vi "Main.vi"() -> ()   [LabVIEW 2017]
doc: "The myRIO Project template acquires acceleration data from the onboard accelerometer and displays the changes of acceleration values in a waveform chart."
uses:
  <vilib>/myRIO/Instrument Drivers/Onboard IO/DIO/typedefs/DIO Reference.ctl
  <vilib>/myRIO/Common/Instrument Driver Framework/Utilities/typedefs/myRIO Generic Hardware Reference.ctl
  <vilib>/myRIO/Common/Instrument Driver Framework/Utilities/typedefs/Hardware Version Enum.ctl
  <vilib>/myRIO/Common/Instrument Driver Framework/Utilities/typedefs/myRIO v1.0 Reference.ctl
  <vilib>/myRIO/Common/Instrument Driver Framework/Utilities/typedefs/Generic FPGA Reference.ctl
  <vilib>/myRIO/Common/Instrument Driver Framework/myRIO v1.0/DIO/typedefs/DIO Channels List.ctl
  <vilib>/myRIO/Common/Instrument Driver Framework/myRIO v1.0/DIO/typedefs/DIO Channels Enum.ctl
  <vilib>/userdefined/High Color/nirio_resource_hc.ctl
  <vilib>/myRIO/Common/Instrument Driver Framework/Utilities/vis/Is FPGA Ref Available.vi
  <vilib>/myRIO/Common/Instrument Driver Framework/myRIO v1.0/DIO/vis/myRIO v1.1 Open DIO.vi
  <vilib>/myRIO/Instrument Drivers/Onboard IO/DIO/vis/Read.vi
  <vilib>/myRIO/Instrument Drivers/Onboard IO/DIO/vis/Write.vi
  <vilib>/myRIO/Common/Instrument Driver Framework/Utilities/vis/Validate Channels.vi
  <vilib>/myRIO/Common/Instrument Driver Framework/myRIO v1.0/DIO/vis/myRIO v1.0 Reserve DIO.vi
  <vilib>/myRIO/Common/Instrument Driver Framework/myRIO v1.0/Resource Manager/vis/myRIO v1.0 Reserve Channel List.vi
  <vilib>/myRIO/Common/Instrument Driver Framework/myRIO v1.0/DIO/vis/myRIO v1.0 Build MUX Configuration DIO.vi
  <vilib>/myRIO/Common/Instrument Driver Framework/myRIO v1.0/Resource Manager/vis/myRIO v1.0 Reserve Channel.vi
  <vilib>/myRIO/Common/Instrument Driver Framework/myRIO v1.0/Resource Manager/vis/myRIO v1.0 Unreserve Channel.vi
  <vilib>/myRIO/Common/Instrument Driver Framework/myRIO v1.0/Resource Manager/vis/myRIO v1.0 Create Configuration List.vi
  <vilib>/myRIO/Common/Instrument Driver Framework/myRIO v1.0/Resource Manager/vis/myRIO v1.0 Build Mutex Name.vi
  GlobalVar.vi
  <vilib>/Utility/VariantDataType/GetNumericInfo.vi
  <vilib>/Utility/error.llb/Error Cluster From Error Code.vi
  <vilib>/myRIO/Common/Instrument Driver Framework/myRIO v1.0/myRIO v1.1 Open.vi
  <vilib>/myRIO/Common/Instrument Driver Framework/Utilities/vis/IO Manager.vi
  <vilib>/myRIO/Common/Instrument Driver Framework/Utilities/vis/Configuration Manager.vi
  <vilib>/myRIO/Common/Instrument Driver Framework/myRIO v1.0/Resource Manager/vis/myRIO v1.0 Configure IO.vi
  <vilib>/myRIO/Common/Instrument Driver Framework/myRIO v1.0/myRIO v1.0 Close.vi
  <vilib>/myRIO/Common/Instrument Driver Framework/myRIO v1.0/DIO/vis/myRIO v1.0 Write DIO.vi
  <vilib>/myRIO/Common/Instrument Driver Framework/myRIO v1.0/DIO/vis/myRIO v1.0 Read DIO.vi
  <vilib>/myRIO/Express VI/Onboard Devices/LED/LED Express VI.xnode
  <vilib>/myRIO/Instrument Drivers/Onboard IO/DIO/vis/myRIO DIO Open.xnode
  <vilib>/myRIO/Express VI/Onboard Devices/Button/Button Express VI.xnode
  <vilib>/myRIO/Instrument Drivers/Onboard IO/DIO/DIO.lvlib
panel:
  out "s? t:f":u32
  in  "servo3 drop_inBack 2":u8
  in  "servo3 pick_front 2":u8=45
  in  "start_seri 2":bool
  in  "done_servo_positioning 2":bool
  in  "inner_b_ir 2":dbl
  in  "inner_f_ir 2":dbl
  in  "target_ir_l 2":dbl
  in  "target_ir_r 2":dbl
  in  "start_cari 2":bool
  in  "done_positioning 2":bool
  in  "servo 3 dropfront 2":u8
  in  "servo 3 pickBack 2":u8
  in  "start_pick 2":bool
  in  "done_pickup 2":bool
  in  "D 2":dbl
  in  "Enum 2":enum16{"hold", "f", "b"}(ring)
  in  "trun 2":bool
  out "binary 2":u32
  out "MOTOR_POW":i8
  in  "Enum":enum16{"hold", "f", "b"}(ring)
  in  "D":dbl
  out "binary":u32
  in  "trun":bool
  in  "servo 3 dropfront":u8
  in  "servo 3 pickBack":u8
  in  "start_pick":bool
  in  "done_pickup":bool
  in  "servo3 pick_front":u8=45
  in  "servo3 drop_inBack":u8
  in  "done_servo_positioning":bool
  in  "start_seri":bool
  in  "inner_f_ir":dbl
  in  "inner_b_ir":dbl
  in  "target_ir_r":dbl
  in  "target_ir_l":dbl
  in  "done_positioning":bool
  in  "start_cari":bool
  in  "x":dbl
  in  "start_step_for_takePic":bool
  in  "Stop (F)":bool
  out "Image Out":T1(plugin-control)
  in  "Carzeta":dbl
  in  "start_rotate_for_takePic":bool
  out "L_MOTOR_POS":i32
  out "R_MOTOR_POS":i32
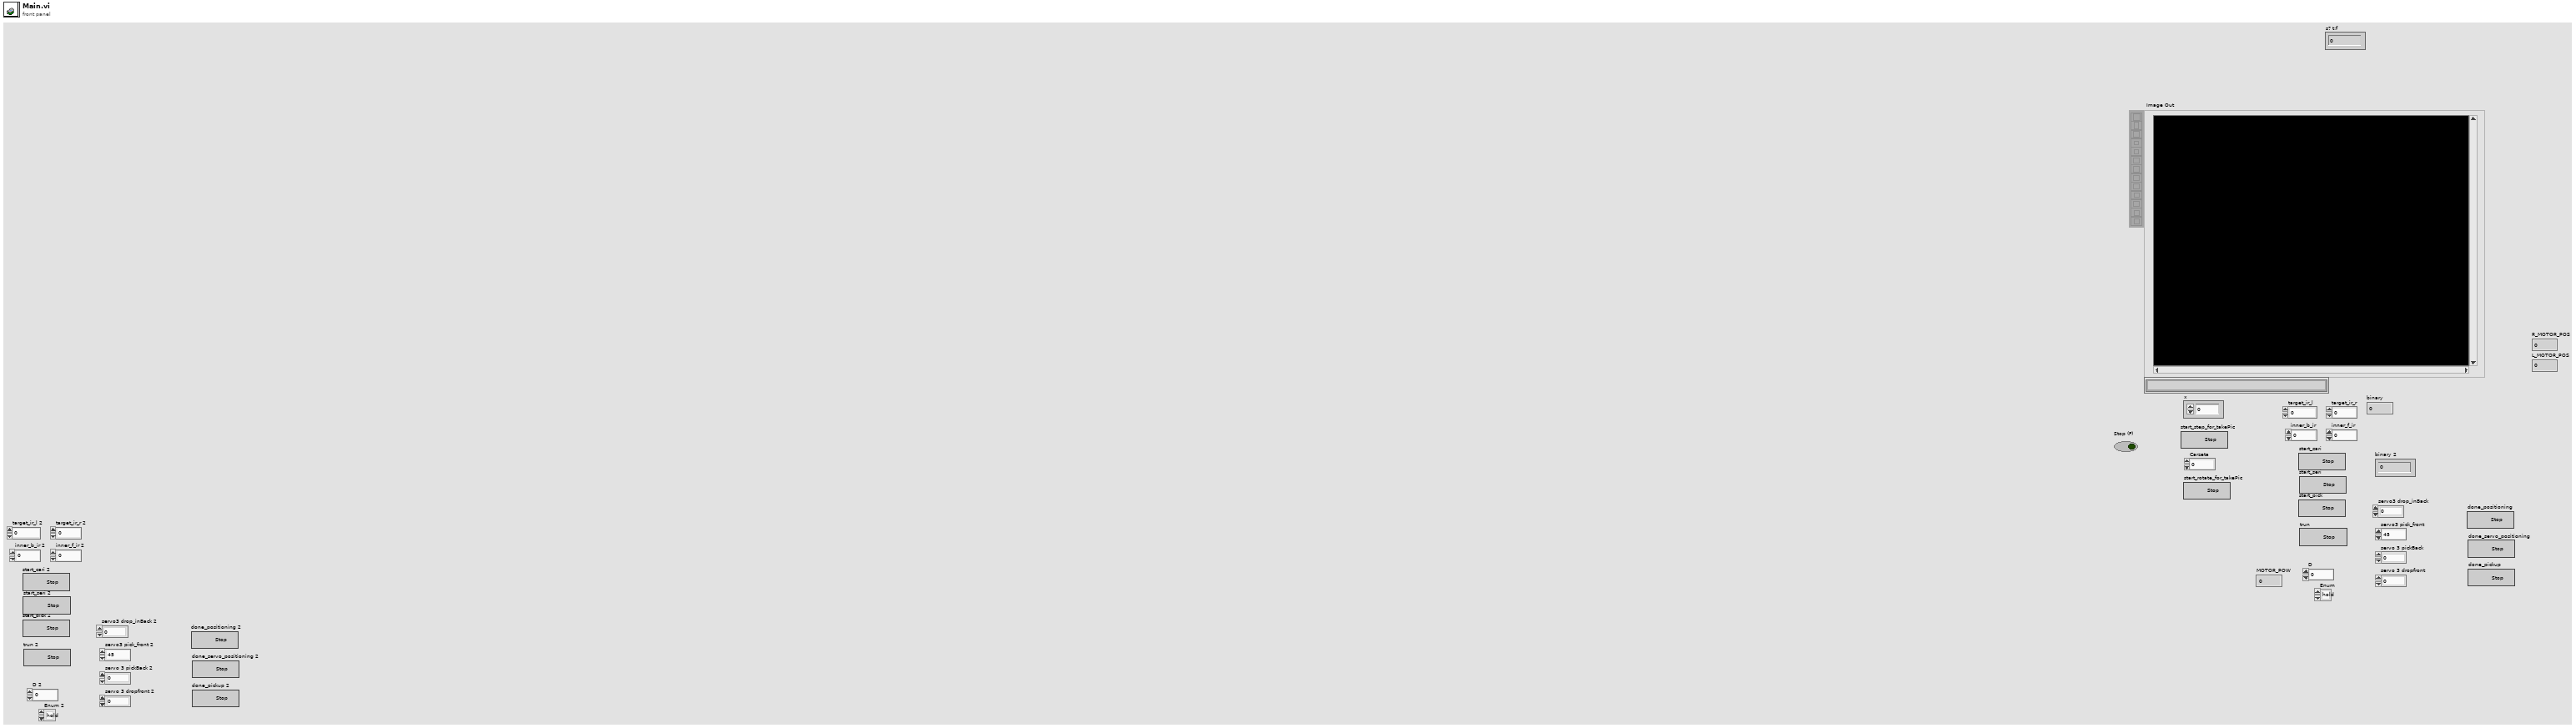
[diagram p1: front panel]
types:
  T1 = typedef "IMAQ Image.ctl" = refnum<image>
  T2 = typedef "DIO.lvlib/DIO Reference.ctl" = cluster{"myRIO Reference":T3, "DIO Channels List":T7}
  T3 = typedef "myRIO Generic Hardware Reference.ctl" = cluster{"myRIO Model":T4, "myRIO Hardware Reference":T5}
  T4 = typedef "Hardware Version Enum.ctl" = enum16{"Unknown", "myRIO-1900", "myRIO-1950", "roboRIO", "NI ELVIS RIO CM"}
  T5 = typedef "myRIO v1.0 Reference.ctl" = cluster{"Generic FPGA Reference":T6, "Allow multiple opens":bool}
  T6 = typedef "Generic FPGA Reference.ctl" = refnum<k20>
  T7 = typedef "DIO Channels List.ctl" = T8[]
  T8 = typedef "DIO Channels Enum.ctl" = enum16{"Not Connected", "C/DIO0", "C/DIO1", "C/DIO2", "C/DIO3", "C/DIO4", "C/DIO5", "C/DIO6", "C/DIO7", "A/DIO0", "A/DIO1", "A/DIO2", "A/DIO3", "A/DIO4", "A/DIO5", "A/DIO6", "A/DIO7", "A/DIO8", "A/DIO9", "A/DIO10", "A/DIO11", "A/DIO12", "A/DIO13", "A/DIO14", "A/DIO15", "B/DIO0", "B/DIO1", "B/DIO2", "B/DIO3", "B/DIO4", "B/DIO5", "B/DIO6", "B/DIO7", "B/DIO8", "B/DIO9", "B/DIO10", "B/DIO11", "B/DIO12", "B/DIO13", "B/DIO14", "B/DIO15", "LED0", "LED1", "LED2", "LED3", "Button0", "DIO/DIO0", "DIO/DIO1", "DIO/DIO2", "DIO/DIO3", "DIO/DIO4", "DIO/DIO5", "DIO/DIO6", "DIO/DIO7", "DIO/DIO8", "DIO/DIO9", "SPI/CS0", "SPI/CS1", "SPI/CS2", "SPI/CS3", "LED RADIO (Green)", "LED RADIO (Red)", "LED COMM (Green)", "LED COMM (Red)", "LED MODE (Green)", "LED MODE (Red)"}
  T9 = typedef "nirio_resource_hc.ctl" = tag
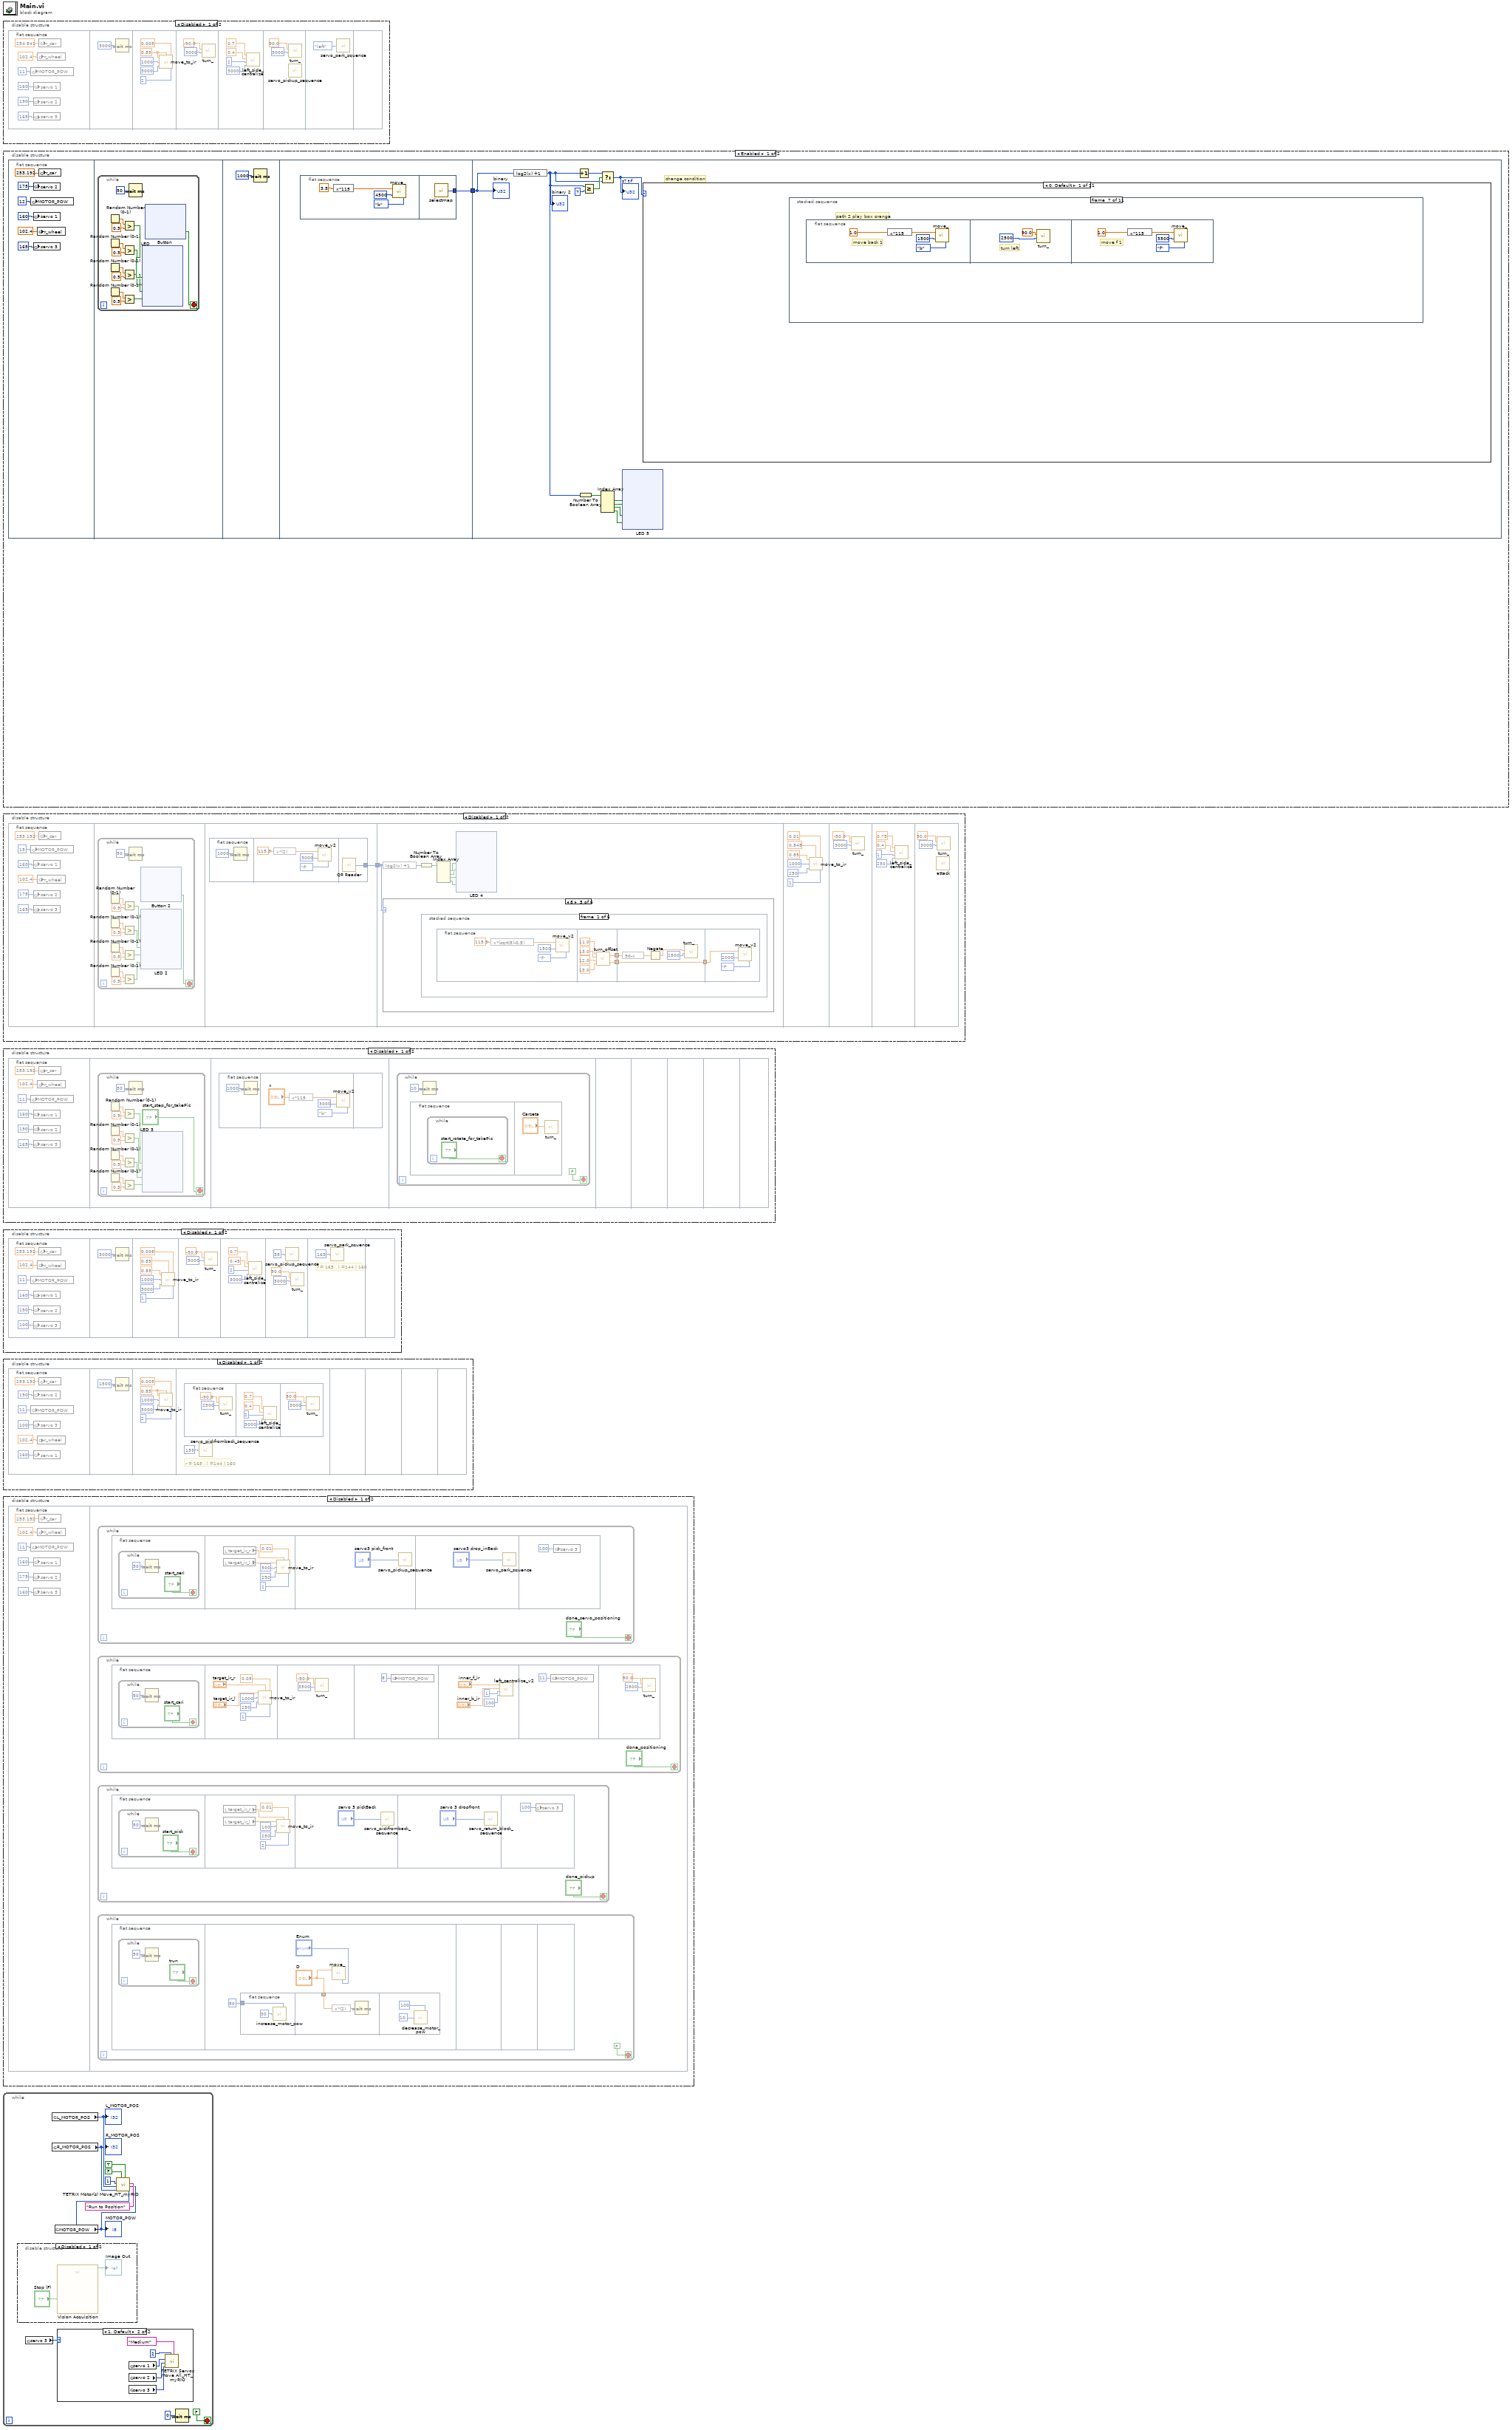
[diagram p0: block diagram]
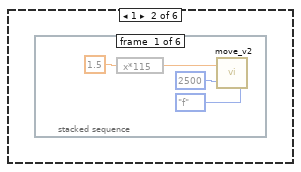
[diagram p5: hidden frame]
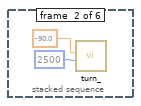
[diagram p6: hidden frame]
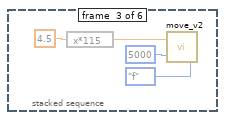
[diagram p7: hidden frame]
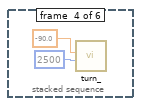
[diagram p8: hidden frame]
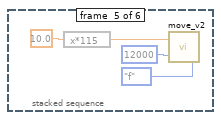
[diagram p9: hidden frame]
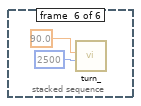
[diagram p10: hidden frame]
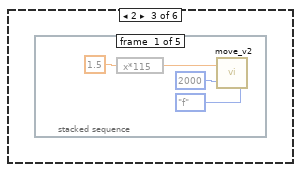
[diagram p11: hidden frame]
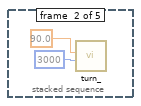
[diagram p12: hidden frame]
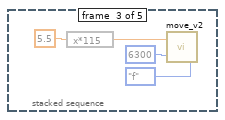
[diagram p13: hidden frame]
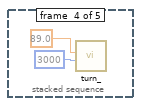
[diagram p14: hidden frame]
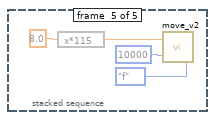
[diagram p15: hidden frame]
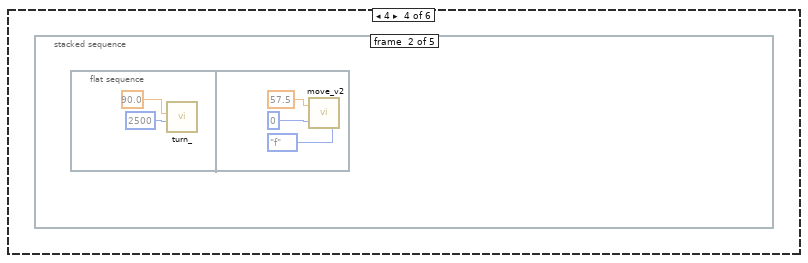
[diagram p16: hidden frame]
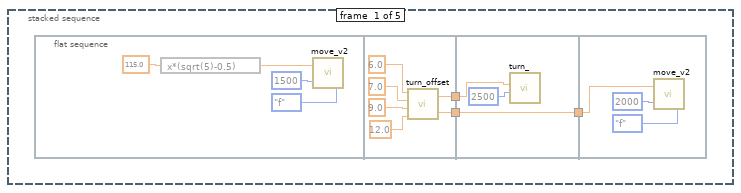
[diagram p17: hidden frame]
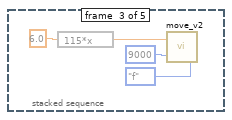
[diagram p18: hidden frame]
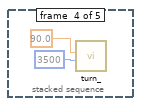
[diagram p19: hidden frame]
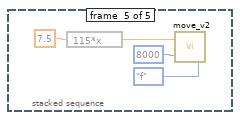
[diagram p20: hidden frame]
diagram:
  n1 = disable-structure shown="Disabled" {
    frame Disabled {
      n2 = flat-sequence {
        frame #0 {
          n3 = global write "GlobalVar.vi" "MOTOR_POW"(i8 11 ("MOTOR_POW")) -> ()
          n4 = global write "GlobalVar.vi" "servo 1"(u8 160 ("servo 1")) -> ()
          n5 = global write "GlobalVar.vi" "servo 2"(u8 190 ("servo 2")) -> ()
          n6 = global write "GlobalVar.vi" "servo 3"(u8 165 ("servo 3")) -> ()
          n7 = global write "GlobalVar.vi" "r_wheel"(102.4 ("r_wheel")) -> ()
          n8 = global write "GlobalVar.vi" "r_car"(254.841 ("r_car")) -> ()
        }
        frame #1 {
          n9 = Wait (ms)(milliseconds to wait=u32 3000) -> ()  [unwired: 1 out]
        }
        frame #2 {
          w12 = 0.85 ("target_ir_r")
          n10 = call "move_to_ir.vi"("step"=2, "precision"=0.005, "target_ir_r"=w12, "samples"=3000, "delay_after"=u32 1000, "target_ir_l"=w12) -> ()
        }
        frame #3 {
          n11 = call "turn_.vi"("delay"=u32 3000, "Carzeta"=-90.0) -> ()  [unwired: 10 in]
        }
        frame #4 {
          n12 = call "left_side_centralize.vi"("samples"=3000, "step(mm)"=2, "inner_b_ir"=0.4, "inner_f_ir"=0.7) -> ()
        }
        frame #5 {
          n13 = call "servo_pickup_sequence.vi"() -> ()  [unwired: 12 in]
          n14 = call "turn_.vi"("delay"=u32 3000, "Carzeta"=90.0) -> ()  [unwired: 10 in]
        }
        frame #6 {
          n15 = call "servo_park_squence.vi"("servo 3"=enum16{"left", "right"}."left" ("pos")) -> ()
        }
        frame #7 {
        }
      }
    }
    frame Enabled {
    }
  }
  n16 = disable-structure shown="Enabled" {
    frame Enabled {
      n17 = flat-sequence {
        tunnel: [w117] -> w22
        tunnel: w22 -> [w128]
        frame #0 {
          n18 = global write "GlobalVar.vi" "MOTOR_POW"(i8 12 ("MOTOR_POW")) -> ()
          n19 = global write "GlobalVar.vi" "servo 2"(u8 175 ("servo 2")) -> ()
          n20 = global write "GlobalVar.vi" "servo 1"(u8 160 ("servo 1")) -> ()
          n21 = global write "GlobalVar.vi" "servo 3"(u8 165 ("servo 3")) -> ()
          n22 = global write "GlobalVar.vi" "r_wheel"(102.4 ("r_wheel")) -> ()
          n23 = global write "GlobalVar.vi" "r_car"(253.192 ("r_car")) -> ()
        }
        frame #1 {
          n24 = while {
            stop <- w29 stop-if-true
            n25 = Random Number (0-1)() -> (number: 0 to 1=w34:dbl)
            n26 = Random Number (0-1)() -> (number: 0 to 1=w41:dbl)
            n27 = Random Number (0-1)() -> (number: 0 to 1=w38:dbl)
            n28 = Random Number (0-1)() -> (number: 0 to 1=w37:dbl)
            n29 = Greater?(x=w34, y=0.5) -> (0:w33:bool)
            n30 = Greater?(x=w41, y=0.5) -> (0:w32:bool)
            n31 = Greater?(x=w38, y=0.5) -> (0:w31:bool)
            n32 = Greater?(x=w37, y=0.5) -> (0:w30:bool)
            n33 = Wait (ms)(milliseconds to wait=u32 50) -> ()  [unwired: 1 out]
            n34 = xnode "LED"("LED0"=w33, "LED1"=w32, "LED2"=w31, "LED3"=w30) -> ()  [unwired: 1 in, 1 out]
            n35 = xnode "Button"() -> ("Value"=w29:bool)  [unwired: 1 in, 1 out]
          }
        }
        frame #2 {
          n36 = Wait (ms)(milliseconds to wait=u32 1000) -> ()  [unwired: 1 out]
        }
        frame #3 {
          n37 = flat-sequence {
            tunnel: [w122] -> w117
            frame #0 {
              n38 = expression code="x*115"(3.5 ("x")) -> (w120:dbl)
              n39 = call "move_.vi"("Enum"=enum16{"hold", "f", "b"}."b", "delay"=u32 4500, "D"=w120) -> ()  [unwired: 1 in]
            }
            frame #1 {
              n40 = call "selectmap.vi"() -> ("binary"=w122:u32)
            }
          }
        }
        frame #4 {
          # "change condition"
          n41 = expression code="log2(x) +1"(w128) -> (w124:u32)
          "binary 2" <- w124
          n42 = Increment(x=w124) -> (x+1=w125:u32)
          n43 = Number To Boolean Array(number=w124) -> (Boolean array=w133:bool[])
          n44 = Greater Or Equal?(x=w124, y=u32 7) -> (x >= y?=w126:bool)
          n45 = Select(t=w125, s=w126, f=w124) -> (s? t:f=w123:u32)
          "s? t:f" <- w123
          n46 = Index Array(array=w133) -> (element #1=w132:bool, element #2=w131:bool, element #3=w130:bool, element #4=w129:bool)  [unwired: 4 in]
          n47 = xnode "LED 5"("LED0"=w132, "LED1"=w131, "LED2"=w130, "LED3"=w129) -> ()  [unwired: 1 in, 1 out]
          n48 = case shown="0, Default" w123 {
            frame 0, Default {
              n49 = stacked-sequence {
                frame #0 {
                  # "font box bule"
                  n50 = flat-sequence {
                    frame #0 {
                      n51 = expression code="x*115"(1.5) -> (w175:dbl)
                      n52 = call "move_.vi"("Enum"=enum16{"hold", "f", "b"}."b", "delay"=u32 2500, "D"=w175) -> ()  [unwired: 1 in]
                    }
                    frame #1 {
                      n53 = call "turn_.vi"("delay"=u32 3000, "Carzeta"=90.0) -> ()  [unwired: 10 in]
                    }
                    frame #2 {
                      n54 = expression code="x*115"(5.0) -> (w181:dbl)
                      n55 = call "move_.vi"("Enum"=enum16{"hold", "f", "b"}."f", "delay"=u32 5500, "D"=w181) -> ()  [unwired: 1 in]
                    }
                    frame #3 {
                      n56 = call "turn_.vi"("delay"=u32 3000, "Carzeta"=-90.0) -> ()  [unwired: 10 in]
                    }
                    frame #4 {
                      n57 = expression code="x*115"(1.0) -> (w187:dbl)
                      n58 = call "move_.vi"("Enum"=enum16{"hold", "f", "b"}."f", "delay"=u32 2500, "D"=w187) -> ()  [unwired: 1 in]
                    }
                    frame #5 {
                      n59 = call "turn_.vi"("delay"=u32 3000, "Carzeta"=90.0) -> ()  [unwired: 10 in]
                    }
                  }
                }
                frame #1 {
                  # "play blue"
                  n60 = flat-sequence {
                    tunnel: [w193] -> w191
                    tunnel: [w192] -> w190
                    tunnel: w191 -> [w198]
                    tunnel: w190 -> [w197]
                    frame #0 {
                      w192 = 0.84 ("target_ir_l")
                      w193 = 0.84 ("target_ir_r")
                      n61 = call "integal_caribat_squence.vi"("inner_b_ir"=0.4, "inner_f_ir"=0.8, "target_ir_l"=w192, "target_ir_r"=w193, "precision"=0.008) -> ()
                    }
                    frame #1 {
                      n62 = call "integal_pickup_sequence .vi"("store_pos"=u8 156, "pick_pos"=u8 52, "target_ir_l"=w197, "target_ir_r"=w198, "precision"=0.05) -> ()
                    }
                  }
                }
                frame #2 {
                  # "move foward 2 box green"
                  n63 = flat-sequence {
                    frame #0 {
                      n64 = call "turn_.vi"("delay"=u32 5000, "Carzeta"=159.44) -> ()  [unwired: 10 in]
                    }
                    frame #1 {
                      n65 = expression code="x*115"(8.54) -> (w205:dbl)
                      n66 = call "move_v2.vi"("delay"=u32 2700, "Enum"=enum16{"hold", "f", "b"}."f", "D"=w205) -> ()  [unwired: 1 in]
                    }
                  }
                }
                frame #3 {
                  # "turn left 2 box green"
                  n67 = flat-sequence {
                    frame #0 {
                      n68 = call "turn_.vi"("delay"=u32 3300, "Carzeta"=110.56) -> ()  [unwired: 10 in]
                    }
                    frame #1 {
                      n69 = expression code="x*115"(8.0) -> (w212:dbl)
                      n70 = call "move_v2.vi"("delay"=u32 2500, "Enum"=enum16{"hold", "f", "b"}."f", "D"=w212) -> ()  [unwired: 1 in]
                    }
                    frame #2 {
                      n71 = call "turn_.vi"("delay"=u32 2500, "Carzeta"=-90.0) -> ()  [unwired: 10 in]
                    }
                  }
                }
                frame #4 {
                  # "play orange 2 right store"
                  n72 = flat-sequence {
                    tunnel: [w219] -> w217
                    tunnel: [w218] -> w216
                    tunnel: w217 -> [w224]
                    tunnel: w216 -> [w223]
                    frame #0 {
                      w218 = 0.84 ("target_ir_l")
                      w219 = 0.84 ("target_ir_r")
                      n73 = call "integal_caribat_squence.vi"("inner_b_ir"=0.4, "inner_f_ir"=0.8, "target_ir_l"=w218, "target_ir_r"=w219, "precision"=0.008) -> ()
                    }
                    frame #1 {
                      n74 = call "integal_pickup_sequence .vi"("store_pos"=u8 183, "pick_pos"=u8 52, "target_ir_l"=w223, "target_ir_r"=w224, "precision"=0.05) -> ()
                    }
                  }
                }
                frame #5 {
                  # "green 2 box green"
                  n75 = call "integal_return.vi"("servo 3 dropfront"=u8 52, "servo 3 pickBack"=u8 154) -> ()
                }
                frame #6 {
                  # "path 2 play box orange"
                  n76 = flat-sequence {
                    frame #0 {
                      # "move back 1"
                      n77 = expression code="x*115"(1.0) -> (w233:dbl)
                      n78 = call "move_.vi"("Enum"=enum16{"hold", "f", "b"}."b", "delay"=u32 1500, "D"=w233) -> ()  [unwired: 1 in]
                    }
                    frame #1 {
                      # "turn left"
                      n79 = call "turn_.vi"("delay"=u32 2500, "Carzeta"=90.0) -> ()  [unwired: 10 in]
                    }
                    frame #2 {
                      # "move f 1"
                      n80 = expression code="x*115"(1.0) -> (w239:dbl)
                      n81 = call "move_.vi"("Enum"=enum16{"hold", "f", "b"}."f", "delay"=u32 3500, "D"=w239) -> ()  [unwired: 1 in]
                    }
                  }
                }
                frame #7 {
                  # "pick red 2 store left"
                  n82 = flat-sequence {
                    tunnel: [w243] -> w241
                    tunnel: [w242] -> w240
                    tunnel: w241 -> [w248]
                    tunnel: w240 -> [w247]
                    frame #0 {
                      w242 = 0.84 ("target_ir_l")
                      w243 = 0.84 ("target_ir_r")
                      n83 = call "integal_caribat_squence.vi"("inner_b_ir"=0.4, "inner_f_ir"=0.8, "target_ir_l"=w242, "target_ir_r"=w243, "precision"=0.008) -> ()
                    }
                    frame #1 {
                      n84 = call "integal_pickup_sequence .vi"("store_pos"=u8 156, "pick_pos"=u8 52, "target_ir_l"=w247, "target_ir_r"=w248, "precision"=0.05) -> ()
                    }
                  }
                }
                frame #8 {
                  # "return orange 2 orange"
                  n85 = call "integal_return.vi"("servo 3 dropfront"=u8 52, "servo 3 pickBack"=u8 183) -> ()
                }
                frame #9 {
                  # "foward 2 parking"
                  n86 = flat-sequence {
                    frame #0 {
                      n87 = call "servo_pickfromback_sequence.vi"("pick_pos"=u8 154) -> ()
                    }
                    frame #1 {
                      n88 = global write "GlobalVar.vi" "servo 3"(u8 30 ("servo 3")) -> ()
                    }
                  }
                  n89 = flat-sequence {
                    frame #0 {
                      n90 = call "turn_.vi"("delay"=u32 5000, "Carzeta"=180.0) -> ()  [unwired: 10 in]
                    }
                    frame #1 {
                      n91 = expression code="x*115"(4.5) -> (w260:dbl)
                      n92 = call "move_.vi"("Enum"=enum16{"hold", "f", "b"}."f", "delay"=u32 5500, "D"=w260) -> ()  [unwired: 1 in]
                    }
                  }
                }
                frame #10 {
                  n93 = flat-sequence {
                    frame #0 {
                      n94 = call "turn_.vi"("delay"=u32 3000, "Carzeta"=-90.0) -> ()  [unwired: 10 in]
                    }
                    frame #1 {
                      n95 = expression code="x*115"(1.5) -> (w266:dbl)
                      n96 = call "move_.vi"("Enum"=enum16{"hold", "f", "b"}."f", "delay"=u32 3000, "D"=w266) -> ()  [unwired: 1 in]
                    }
                  }
                }
              }
            }
            frame 1 {
              n97 = stacked-sequence {
                frame #0 {
                  # "out parking"
                  n98 = flat-sequence {
                    tunnel: [w272] -> w270
                    tunnel: [w271] -> w268
                    tunnel: w270 -> [w279]
                    tunnel: [w278] -> w269
                    tunnel: w268 -> [w278]
                    tunnel: w269 -> [w281]
                    frame #0 {
                      n99 = call "turn_offset.vi"("x2"=17.0, "x1"=16.0, "y2"=16.0, "y1"=13.0) -> ("dis_"=w271:dbl, "zeta"=w272:dbl)
                    }
                    frame #1 {
                      n100 = expression code="-(45-x)"(w279) -> (w277:dbl)
                      n101 = call "turn_.vi"("delay"=u32 3000, "Carzeta"=w277) -> ()  [unwired: 10 in]
                    }
                    frame #2 {
                      n102 = call "move_.vi"("Enum"=enum16{"hold", "f", "b"}."b", "delay"=u32 2000, "D"=w281) -> ()  [unwired: 1 in]
                    }
                  }
                }
                frame #1 {
                  # "path 2 box blue"
                  n103 = flat-sequence {
                    frame #0 {
                      n104 = call "turn_.vi"("delay"=u32 3000, "Carzeta"=-90.0) -> ()  [unwired: 10 in]
                    }
                    frame #1 {
                      # "foward 2 blue"
                      n105 = expression code="x*115"(6.0) -> (w288:dbl)
                      n106 = call "move_.vi"("Enum"=enum16{"hold", "f", "b"}."f", "delay"=u32 6500, "D"=w288) -> ()  [unwired: 1 in]
                    }
                    frame #2 {
                      # "turn left"
                      n107 = call "turn_.vi"("delay"=u32 3000, "Carzeta"=90.0) -> ()  [unwired: 10 in]
                    }
                    frame #3 {
                      # "foward 2 blue"
                      n108 = expression code="x*115"(1.0) -> (w294:dbl)
                      n109 = call "move_.vi"("Enum"=enum16{"hold", "f", "b"}."f", "delay"=u32 1500, "D"=w294) -> ()  [unwired: 1 in]
                    }
                    frame #4 {
                      # "turn right"
                      n110 = call "turn_.vi"("delay"=u32 3000, "Carzeta"=-90.0) -> ()  [unwired: 10 in]
                    }
                  }
                }
                frame #2 {
                  # "keep yellow 2 left stored"
                  n111 = flat-sequence {
                    tunnel: [w301] -> w299
                    tunnel: [w300] -> w298
                    tunnel: w299 -> [w306]
                    tunnel: w298 -> [w305]
                    frame #0 {
                      w300 = 0.84 ("target_ir_l")
                      w301 = 0.84 ("target_ir_r")
                      n112 = call "integal_caribat_squence.vi"("inner_b_ir"=0.4, "inner_f_ir"=0.8, "target_ir_l"=w300, "target_ir_r"=w301, "precision"=0.008) -> ()
                    }
                    frame #1 {
                      n113 = call "integal_pickup_sequence .vi"("store_pos"=u8 156, "pick_pos"=u8 52, "target_ir_l"=w305, "target_ir_r"=w306, "precision"=0.05) -> ()
                    }
                  }
                }
                frame #3 {
                  # "path 2 box yellow(1)"
                  n114 = flat-sequence {
                    frame #0 {
                      # "turn right"
                      n115 = call "turn_.vi"("delay"=u32 5000, "Carzeta"=-142.125) -> ()  [unwired: 10 in]
                    }
                    frame #1 {
                      # "foward 2 yellow"
                      n116 = expression code="x*115"(11.4) -> (w313:dbl)
                      n117 = call "move_v2.vi"("delay"=u32 3500, "Enum"=enum16{"hold", "f", "b"}."f", "D"=w313) -> ()  [unwired: 1 in]
                    }
                    frame #2 {
                      # "turn right"
                      n118 = call "turn_.vi"("delay"=u32 2000, "Carzeta"=-37.875) -> ()  [unwired: 10 in]
                    }
                  }
                }
                frame #4 {
                  # "green 2 right stored"
                  n119 = flat-sequence {
                    tunnel: [w321] -> w319
                    tunnel: [w320] -> w318
                    tunnel: w319 -> [w326]
                    tunnel: w318 -> [w325]
                    frame #0 {
                      w320 = 0.84 ("target_ir_l")
                      w321 = 0.84 ("target_ir_r")
                      n120 = call "integal_caribat_squence.vi"("inner_b_ir"=0.4, "inner_f_ir"=0.8, "target_ir_l"=w320, "target_ir_r"=w321, "precision"=0.008) -> ()
                    }
                    frame #1 {
                      n121 = call "integal_pickup_sequence .vi"("store_pos"=u8 183, "pick_pos"=u8 52, "target_ir_l"=w325, "target_ir_r"=w326, "precision"=0.04) -> ()
                    }
                  }
                }
                frame #5 {
                  # "yellow 2 yellow"
                  # "154"
                  n122 = call "integal_return.vi"("servo 3 dropfront"=u8 52, "servo 3 pickBack"=u8 154) -> ()
                }
                frame #6 {
                  # "path 2 box green (1)"
                  n123 = flat-sequence {
                    frame #0 {
                      # "turn right"
                      n124 = call "turn_.vi"("delay"=u32 3000, "Carzeta"=-90.0) -> ()  [unwired: 10 in]
                    }
                    frame #1 {
                      # "forward 2 g"
                      n125 = expression code="x*115"(2.0) -> (w336:dbl)
                      n126 = call "move_.vi"("Enum"=enum16{"hold", "f", "b"}."f", "delay"=u32 2500, "D"=w336) -> ()  [unwired: 1 in]
                    }
                  }
                }
                frame #7 {
                  # "path 2 box green (2)"
                  n127 = flat-sequence {
                    frame #0 {
                      # "turn right"
                      n128 = call "turn_.vi"("delay"=u32 3000, "Carzeta"=-90.0) -> ()  [unwired: 10 in]
                    }
                    frame #1 {
                      # "foward 2 green"
                      n129 = expression code="x*115"(9.0) -> (w341:dbl)
                      n130 = call "move_v2.vi"("delay"=u32 3000, "Enum"=enum16{"hold", "f", "b"}."f", "D"=w341) -> ()  [unwired: 1 in]
                    }
                    frame #2 {
                      n131 = call "turn_.vi"("delay"=u32 3000, "Carzeta"=-90.0) -> ()  [unwired: 10 in]
                    }
                  }
                }
                frame #8 {
                  # "red 2 stored left"
                  n132 = flat-sequence {
                    tunnel: [w355] -> w347
                    tunnel: [w354] -> w346
                    tunnel: w347 -> [w360]
                    tunnel: w346 -> [w359]
                    frame #0 {
                      w354 = 0.84 ("target_ir_l")
                      w355 = 0.84 ("target_ir_r")
                      n133 = call "integal_caribat_squence.vi"("inner_b_ir"=0.4, "inner_f_ir"=0.8, "target_ir_l"=w354, "target_ir_r"=w355, "precision"=0.008) -> ()
                    }
                    frame #1 {
                      n134 = call "integal_pickup_sequence .vi"("store_pos"=u8 156, "pick_pos"=u8 52, "target_ir_l"=w359, "target_ir_r"=w360, "precision"=0.04) -> ()
                    }
                  }
                  n135 = disable-structure shown="Disabled" {
                    frame Disabled {
                      n136 = flat-sequence {
                        frame #0 {
                          n137 = call "integal_caribat_squence.vi"("inner_b_ir"=0.4, "inner_f_ir"=0.8, "target_ir_l"=0.84, "target_ir_r"=0.84, "precision"=0.008) -> ()
                        }
                        frame #1 {
                          n138 = call "servo_return_block_sequence.vi"("servo 3"=u8 52) -> ()
                        }
                      }
                    }
                    frame Enabled {
                    }
                  }
                }
                frame #9 {
                  # "path 2 parking"
                  n139 = flat-sequence {
                    frame #0 {
                      n140 = call "servo_pickfromback_sequence.vi"("pick_pos"=u8 182) -> ()
                    }
                    frame #1 {
                      n141 = global write "GlobalVar.vi" "servo 3"(u8 52 ("servo 3")) -> ()
                    }
                  }
                  n142 = flat-sequence {
                    frame #0 {
                      n143 = call "turn_.vi"("delay"=u32 3000, "Carzeta"=-90.0) -> ()  [unwired: 10 in]
                    }
                    frame #1 {
                      n144 = expression code="x*115"(7.0) -> (w370:dbl)
                      n145 = call "move_v2.vi"("delay"=u32 2300, "Enum"=enum16{"hold", "f", "b"}."f", "D"=w370) -> ()  [unwired: 1 in]
                    }
                    frame #2 {
                      n146 = call "turn_.vi"("delay"=u32 3000, "Carzeta"=-90.0) -> ()  [unwired: 10 in]
                    }
                    frame #3 {
                      n147 = expression code="x*115"(5.0) -> (w376:dbl)
                      n148 = call "move_.vi"("Enum"=enum16{"hold", "f", "b"}."f", "delay"=u32 4500, "D"=w376) -> ()  [unwired: 1 in]
                    }
                  }
                }
              }
            }
            frame 2 {
              n149 = stacked-sequence {
                frame #0 {
                  # "out parking"
                  n150 = flat-sequence {
                    tunnel: [w382] -> w380
                    tunnel: [w381] -> w378
                    tunnel: w380 -> [w389]
                    tunnel: [w388] -> w379
                    tunnel: w378 -> [w388]
                    tunnel: w379 -> [w391]
                    frame #0 {
                      n151 = call "turn_offset.vi"("x2"=5.0, "x1"=7.0, "y2"=9.0, "y1"=8.0) -> ("dis_"=w381:dbl, "zeta"=w382:dbl)
                    }
                    frame #1 {
                      n152 = expression code="-45-x"(w389) -> (w387:dbl)
                      n153 = call "turn_.vi"("delay"=u32 3000, "Carzeta"=w387) -> ()  [unwired: 10 in]
                    }
                    frame #2 {
                      n154 = call "move_.vi"("Enum"=enum16{"hold", "f", "b"}."b", "delay"=u32 2000, "D"=w391) -> ()  [unwired: 1 in]
                    }
                  }
                }
                frame #1 {
                  # "path 2 box green"
                  n155 = flat-sequence {
                    frame #0 {
                      # "turn left"
                      n156 = call "turn_.vi"("delay"=u32 3000, "Carzeta"=90.0) -> ()  [unwired: 10 in]
                    }
                    frame #1 {
                      n157 = expression code="x*115"(1.0) -> (w398:dbl)
                      n158 = call "move_.vi"("Enum"=enum16{"hold", "f", "b"}."b", "delay"=u32 3500, "D"=w398) -> ()  [unwired: 1 in]
                    }
                    frame #2 {
                      n159 = call "turn_.vi"("delay"=u32 3000, "Carzeta"=90.0) -> ()  [unwired: 10 in]
                    }
                    frame #3 {
                      # "foward 2 yellow"
                      n160 = expression code="x*115"(8.0) -> (w403:dbl)
                      n161 = call "move_v2.vi"("delay"=u32 2000, "Enum"=enum16{"hold", "f", "b"}."f", "D"=w403) -> ()  [unwired: 1 in]
                    }
                  }
                }
                frame #2 {
                  # "keep orange 2 left stored"
                  n162 = flat-sequence {
                    tunnel: [w409] -> w407
                    tunnel: [w408] -> w406
                    tunnel: w407 -> [w414]
                    tunnel: w406 -> [w413]
                    frame #0 {
                      w408 = 0.84 ("target_ir_l")
                      w409 = 0.84 ("target_ir_r")
                      n163 = call "integal_caribat_squence.vi"("inner_b_ir"=0.4, "inner_f_ir"=0.8, "target_ir_l"=w408, "target_ir_r"=w409, "precision"=0.008) -> ()
                    }
                    frame #1 {
                      n164 = call "integal_pickup_sequence .vi"("store_pos"=u8 156, "pick_pos"=u8 52, "target_ir_l"=w413, "target_ir_r"=w414, "precision"=0.05) -> ()
                    }
                  }
                }
                frame #3 {
                  # "path 2 box orange(1)"
                  n165 = flat-sequence {
                    frame #0 {
                      n166 = expression code="x*115"(2.0) -> (w420:dbl)
                      n167 = call "move_.vi"("Enum"=enum16{"hold", "f", "b"}."b", "delay"=u32 3500, "D"=w420) -> ()  [unwired: 1 in]
                    }
                    frame #1 {
                      # "turn left 2 yellow"
                      n168 = call "turn_.vi"("delay"=u32 3000, "Carzeta"=90.0) -> ()  [unwired: 10 in]
                    }
                    frame #2 {
                      # "foward 2 orange"
                      n169 = expression code="x*115"(7.0) -> (w427:dbl)
                      n170 = call "move_v2.vi"("delay"=u32 3000, "Enum"=enum16{"hold", "f", "b"}."f", "D"=w427) -> ()  [unwired: 1 in]
                    }
                  }
                }
                frame #4 {
                  # "red 2 right stored"
                  n171 = flat-sequence {
                    tunnel: [w431] -> w429
                    tunnel: [w430] -> w428
                    tunnel: w429 -> [w436]
                    tunnel: w428 -> [w435]
                    frame #0 {
                      w430 = 0.84 ("target_ir_l")
                      w431 = 0.84 ("target_ir_r")
                      n172 = call "integal_caribat_squence.vi"("inner_b_ir"=0.4, "inner_f_ir"=0.8, "target_ir_l"=w430, "target_ir_r"=w431, "precision"=0.008) -> ()
                    }
                    frame #1 {
                      n173 = call "integal_pickup_sequence .vi"("store_pos"=u8 183, "pick_pos"=u8 52, "target_ir_l"=w435, "target_ir_r"=w436, "precision"=0.04) -> ()
                    }
                  }
                }
                frame #5 {
                  # "orange 2 orange"
                  # "154"
                  n174 = call "integal_return.vi"("servo 3 dropfront"=u8 52, "servo 3 pickBack"=u8 154) -> ()
                }
                frame #6 {
                  # "path 2 box blue (1)"
                  n175 = flat-sequence {
                    frame #0 {
                      # "forward 2 g"
                      n176 = expression code="x*115"(1.0) -> (w444:dbl)
                      n177 = call "move_.vi"("Enum"=enum16{"hold", "f", "b"}."b", "delay"=u32 2500, "D"=w444) -> ()  [unwired: 1 in]
                    }
                    frame #1 {
                      # "turn left"
                      n178 = call "turn_.vi"("delay"=u32 3000, "Carzeta"=90.0) -> ()  [unwired: 10 in]
                    }
                    frame #2 {
                      # "forward 2 g"
                      n179 = expression code="x*115"(5.0) -> (w451:dbl)
                      n180 = call "move_.vi"("Enum"=enum16{"hold", "f", "b"}."f", "delay"=u32 5500, "D"=w451) -> ()  [unwired: 1 in]
                    }
                    frame #3 {
                      n181 = call "turn_.vi"("delay"=u32 3000, "Carzeta"=-90.0) -> ()  [unwired: 10 in]
                    }
                  }
                }
                frame #7 {
                  # "need turn"
                  # "green 2 stored left"
                  n182 = flat-sequence {
                    tunnel: [w463] -> w455
                    tunnel: [w462] -> w454
                    tunnel: w455 -> [w468]
                    tunnel: w454 -> [w467]
                    frame #0 {
                      w462 = 0.84 ("target_ir_l")
                      w463 = 0.84 ("target_ir_r")
                      n183 = call "integal_caribat_squence.vi"("inner_b_ir"=0.4, "inner_f_ir"=0.8, "target_ir_l"=w462, "target_ir_r"=w463, "precision"=0.008) -> ()
                    }
                    frame #1 {
                      n184 = call "integal_pickup_sequence .vi"("store_pos"=u8 156, "pick_pos"=u8 52, "target_ir_l"=w467, "target_ir_r"=w468, "precision"=0.05) -> ()
                    }
                  }
                  n185 = disable-structure shown="Disabled" {
                    frame Disabled {
                      n186 = flat-sequence {
                        frame #0 {
                          n187 = call "integal_caribat_squence.vi"("inner_b_ir"=0.4, "inner_f_ir"=0.8, "target_ir_l"=0.84, "target_ir_r"=0.84, "precision"=0.008) -> ()
                        }
                        frame #1 {
                          n188 = call "servo_return_block_sequence.vi"("servo 3"=u8 52) -> ()
                        }
                      }
                    }
                    frame Enabled {
                    }
                  }
                }
                frame #8 {
                  # "back 2 green"
                  n189 = flat-sequence {
                    frame #0 {
                      # "forward 2 g"
                      n190 = expression code="x*115"(6.0) -> (w474:dbl)
                      n191 = call "move_.vi"("Enum"=enum16{"hold", "f", "b"}."b", "delay"=u32 7000, "D"=w474) -> ()  [unwired: 1 in]
                    }
                    frame #1 {
                      # "turn right"
                      n192 = call "turn_.vi"("delay"=u32 3000, "Carzeta"=-90.0) -> ()  [unwired: 10 in]
                    }
                    frame #2 {
                      n193 = expression code="x*115"(7.0) -> (w481:dbl)
                      n194 = call "move_v2.vi"("delay"=u32 2300, "Enum"=enum16{"hold", "f", "b"}."f", "D"=w481) -> ()  [unwired: 1 in]
                    }
                  }
                }
                frame #9 {
                  # "154"
                  # "return green 2 geen"
                  n195 = call "integal_return.vi"("servo 3 dropfront"=u8 52, "servo 3 pickBack"=u8 154) -> ()
                }
                frame #10 {
                  n196 = flat-sequence {
                    frame #0 {
                      n197 = call "servo_pickfromback_sequence.vi"("pick_pos"=u8 182) -> ()
                    }
                    frame #1 {
                      n198 = global write "GlobalVar.vi" "servo 3"(u8 52 ("servo 3")) -> ()
                    }
                  }
                  n199 = flat-sequence {
                    frame #0 {
                      n200 = call "turn_.vi"("delay"=u32 5000, "Carzeta"=180.0) -> ()  [unwired: 10 in]
                    }
                    frame #1 {
                      n201 = expression code="x*115"(9.0) -> (w490:dbl)
                      n202 = call "move_v2.vi"("delay"=u32 3000, "Enum"=enum16{"hold", "f", "b"}."f", "D"=w490) -> ()  [unwired: 1 in]
                    }
                    frame #2 {
                      n203 = call "turn_.vi"("delay"=u32 3000, "Carzeta"=90.0) -> ()  [unwired: 10 in]
                    }
                    frame #3 {
                      n204 = expression code="x*115"(0.5) -> (w496:dbl)
                      n205 = call "move_.vi"("Enum"=enum16{"hold", "f", "b"}."f", "delay"=u32 1000, "D"=w496) -> ()  [unwired: 1 in]
                    }
                    frame #4 {
                      n206 = call "turn_offset.vi"("x2"=5.0, "x1"=7.0, "y2"=9.0, "y1"=8.0) -> ("zeta"=w499:dbl)  [unwired: 1 out]
                      n207 = expression code="90-x"(w499) -> (w498:dbl)
                      n208 = call "turn_.vi"("delay"=u32 3000, "Carzeta"=w498) -> ()  [unwired: 10 in]
                    }
                    frame #5 {
                      n209 = expression code="x*115"(1.0) -> (w507:dbl)
                      n210 = call "move_.vi"("Enum"=enum16{"hold", "f", "b"}."f", "delay"=u32 1500, "D"=w507) -> ()  [unwired: 1 in]
                    }
                  }
                }
              }
            }
            frame 3 {
              n211 = stacked-sequence {
                frame #0 {
                  # "out parking"
                  n212 = flat-sequence {
                    tunnel: [w513] -> w511
                    tunnel: [w512] -> w509
                    tunnel: w511 -> [w520]
                    tunnel: [w519] -> w510
                    tunnel: w509 -> [w519]
                    tunnel: w510 -> [w522]
                    frame #0 {
                      n213 = call "turn_offset.vi"("x2"=17.0, "x1"=15.0, "y2"=13.0, "y1"=12.0) -> ("dis_"=w512:dbl, "zeta"=w513:dbl)
                    }
                    frame #1 {
                      n214 = expression code="45+x"(w520) -> (w518:dbl)
                      n215 = call "turn_.vi"("delay"=u32 3000, "Carzeta"=w518) -> ()  [unwired: 10 in]
                    }
                    frame #2 {
                      n216 = call "move_.vi"("Enum"=enum16{"hold", "f", "b"}."b", "delay"=u32 2000, "D"=w522) -> ()  [unwired: 1 in]
                    }
                  }
                }
                frame #1 {
                  # "path 2 box blue"
                  n217 = flat-sequence {
                    frame #0 {
                      # "turn left"
                      n218 = call "turn_.vi"("delay"=u32 5000, "Carzeta"=180.0) -> ()  [unwired: 10 in]
                    }
                    frame #1 {
                      # "forward 2 g"
                      n219 = expression code="x*115"(4.0) -> (w530:dbl)
                      n220 = call "move_.vi"("Enum"=enum16{"hold", "f", "b"}."f", "delay"=u32 4500, "D"=w530) -> ()  [unwired: 1 in]
                    }
                    frame #2 {
                      # "turn left"
                      n221 = call "turn_.vi"("delay"=u32 3000, "Carzeta"=90.0) -> ()  [unwired: 10 in]
                    }
                    frame #3 {
                      # "forward 2 g"
                      n222 = expression code="x*115"(3.0) -> (w536:dbl)
                      n223 = call "move_.vi"("Enum"=enum16{"hold", "f", "b"}."f", "delay"=u32 3500, "D"=w536) -> ()  [unwired: 1 in]
                    }
                    frame #4 {
                      # "turn left"
                      n224 = call "turn_.vi"("delay"=u32 3000, "Carzeta"=-90.0) -> ()  [unwired: 10 in]
                    }
                  }
                }
                frame #2 {
                  # "keep yellow 2 left stored"
                  n225 = flat-sequence {
                    tunnel: [w542] -> w540
                    tunnel: [w541] -> w539
                    tunnel: w540 -> [w547]
                    tunnel: w539 -> [w546]
                    frame #0 {
                      w541 = 0.84 ("target_ir_l")
                      w542 = 0.84 ("target_ir_r")
                      n226 = call "integal_caribat_squence.vi"("inner_b_ir"=0.4, "inner_f_ir"=0.8, "target_ir_l"=w541, "target_ir_r"=w542, "precision"=0.008) -> ()
                    }
                    frame #1 {
                      n227 = call "integal_pickup_sequence .vi"("store_pos"=u8 156, "pick_pos"=u8 52, "target_ir_l"=w546, "target_ir_r"=w547, "precision"=0.05) -> ()
                    }
                  }
                }
                frame #3 {
                  # "path 2 box yellow(1)"
                  n228 = flat-sequence {
                    frame #0 {
                      n229 = call "turn_.vi"("delay"=u32 3000, "Carzeta"=-90.0) -> ()  [unwired: 10 in]
                    }
                    frame #1 {
                      n230 = expression code="x*115"(7.0) -> (w556:dbl)
                      n231 = call "move_v2.vi"("delay"=u32 3000, "Enum"=enum16{"hold", "f", "b"}."f", "D"=w556) -> ()  [unwired: 1 in]
                    }
                    frame #2 {
                      # "turn right 2 yellow"
                      n232 = call "turn_.vi"("delay"=u32 3000, "Carzeta"=-90.0) -> ()  [unwired: 10 in]
                    }
                    frame #3 {
                      # "foward 2 yellow"
                      n233 = expression code="x*115"(7.0) -> (w562:dbl)
                      n234 = call "move_v2.vi"("delay"=u32 2000, "Enum"=enum16{"hold", "f", "b"}."f", "D"=w562) -> ()  [unwired: 1 in]
                    }
                  }
                }
                frame #4 {
                  # "green 2 right stored"
                  n235 = flat-sequence {
                    tunnel: [w566] -> w564
                    tunnel: [w565] -> w563
                    tunnel: w564 -> [w571]
                    tunnel: w563 -> [w570]
                    frame #0 {
                      w565 = 0.84 ("target_ir_l")
                      w566 = 0.84 ("target_ir_r")
                      n236 = call "integal_caribat_squence.vi"("inner_b_ir"=0.4, "inner_f_ir"=0.8, "target_ir_l"=w565, "target_ir_r"=w566, "precision"=0.008) -> ()
                    }
                    frame #1 {
                      n237 = call "integal_pickup_sequence .vi"("store_pos"=u8 183, "pick_pos"=u8 52, "target_ir_l"=w570, "target_ir_r"=w571, "precision"=0.05) -> ()
                    }
                  }
                }
                frame #5 {
                  # "return yellow"
                  # "154"
                  n238 = call "integal_return.vi"("servo 3 dropfront"=u8 52, "servo 3 pickBack"=u8 154) -> ()
                }
                frame #6 {
                  # "path 2 box green (1)"
                  n239 = flat-sequence {
                    frame #0 {
                      # "forward 2 g"
                      n240 = expression code="x*115"(2.0) -> (w579:dbl)
                      n241 = call "move_.vi"("Enum"=enum16{"hold", "f", "b"}."b", "delay"=u32 2500, "D"=w579) -> ()  [unwired: 1 in]
                    }
                    frame #1 {
                      # "turn left"
                      n242 = call "turn_.vi"("delay"=u32 3000, "Carzeta"=90.0) -> ()  [unwired: 10 in]
                    }
                  }
                }
                frame #7 {
                  # "red 2 stored left"
                  n243 = flat-sequence {
                    tunnel: [w592] -> w584
                    tunnel: [w591] -> w583
                    tunnel: w584 -> [w597]
                    tunnel: w583 -> [w596]
                    frame #0 {
                      w591 = 0.84 ("target_ir_l")
                      w592 = 0.84 ("target_ir_r")
                      n244 = call "integal_caribat_squence.vi"("inner_b_ir"=0.4, "inner_f_ir"=0.8, "target_ir_l"=w591, "target_ir_r"=w592, "precision"=0.008) -> ()
                    }
                    frame #1 {
                      n245 = call "integal_pickup_sequence .vi"("store_pos"=u8 156, "pick_pos"=u8 52, "target_ir_l"=w596, "target_ir_r"=w597, "precision"=0.04) -> ()
                    }
                  }
                  n246 = disable-structure shown="Disabled" {
                    frame Disabled {
                      n247 = flat-sequence {
                        frame #0 {
                          n248 = call "integal_caribat_squence.vi"("inner_b_ir"=0.4, "inner_f_ir"=0.8, "target_ir_l"=0.84, "target_ir_r"=0.84, "precision"=0.008) -> ()
                        }
                        frame #1 {
                          n249 = call "servo_return_block_sequence.vi"("servo 3"=u8 52) -> ()
                        }
                      }
                    }
                    frame Enabled {
                    }
                  }
                }
                frame #8 {
                  # "154"
                  # "return green 2 geen"
                  n250 = call "integal_return.vi"("servo 3 dropfront"=u8 52, "servo 3 pickBack"=u8 183) -> ()
                }
                frame #9 {
                  # "path 2 parking"
                  n251 = flat-sequence {
                    frame #0 {
                      n252 = call "servo_pickfromback_sequence.vi"("pick_pos"=u8 156) -> ()
                    }
                    frame #1 {
                      n253 = global write "GlobalVar.vi" "servo 3"(u8 34 ("servo 3")) -> ()
                    }
                  }
                  n254 = flat-sequence {
                    frame #0 {
                      n255 = call "turn_.vi"("delay"=u32 4500, "Carzeta"=158.198) -> ()  [unwired: 10 in]
                    }
                    frame #1 {
                      n256 = expression code="x*115"(5.385) -> (w609:dbl)
                      n257 = call "move_v2.vi"("delay"=u32 3000, "Enum"=enum16{"hold", "f", "b"}."f", "D"=w609) -> ()  [unwired: 1 in]
                    }
                  }
                }
                frame #10 {
                  n258 = flat-sequence {
                    frame #0 {
                      n259 = call "turn_.vi"("delay"=u32 3000, "Carzeta"=90.0) -> ()  [unwired: 10 in]
                    }
                    frame #1 {
                      n260 = expression code="x*115"(1.5) -> (w616:dbl)
                      n261 = call "move_.vi"("Enum"=enum16{"hold", "f", "b"}."f", "delay"=u32 2500, "D"=w616) -> ()  [unwired: 1 in]
                    }
                  }
                }
              }
            }
            frame 4 {
              n262 = stacked-sequence {
                frame #0 {
                  n263 = flat-sequence {
                    tunnel: [w621] -> w619
                    tunnel: [w620] -> w618
                    tunnel: w619 -> [w628]
                    tunnel: [w627] -> w617
                    tunnel: w618 -> [w627]
                    tunnel: w617 -> [w630]
                    frame #0 {
                      n264 = call "turn_offset.vi"("x2"=13.0, "x1"=15.0, "y2"=17.0, "y1"=16.0) -> ("dis_"=w620:dbl, "zeta"=w621:dbl)
                    }
                    frame #1 {
                      n265 = expression code="45-x"(w628) -> (w626:dbl)
                      n266 = call "turn_.vi"("delay"=u32 3000, "Carzeta"=w626) -> ()  [unwired: 10 in]
                    }
                    frame #2 {
                      n267 = call "move_.vi"("Enum"=enum16{"hold", "f", "b"}."b", "delay"=u32 2000, "D"=w630) -> ()  [unwired: 1 in]
                    }
                  }
                }
                frame #1 {
                  n268 = flat-sequence {
                    frame #0 {
                      n269 = call "turn_.vi"("delay"=u32 3000, "Carzeta"=-158.16) -> ()  [unwired: 10 in]
                    }
                    frame #1 {
                      n270 = expression code="x*115"(5.385) -> (w638:dbl)
                      n271 = call "move_.vi"("Enum"=enum16{"hold", "f", "b"}."f", "delay"=u32 6500, "D"=w638) -> ()  [unwired: 1 in]
                    }
                  }
                }
                frame #2 {
                  n272 = flat-sequence {
                    frame #0 {
                      n273 = call "turn_.vi"("delay"=u32 3000, "Carzeta"=-111.8) -> ()  [unwired: 10 in]
                    }
                    frame #1 {
                      n274 = expression code="x*115"(1.0) -> (w644:dbl)
                      n275 = call "move_.vi"("Enum"=enum16{"hold", "f", "b"}."f", "delay"=u32 1500, "D"=w644) -> ()  [unwired: 1 in]
                    }
                  }
                }
                frame #3 {
                  n276 = flat-sequence {
                    tunnel: [w648] -> w646
                    tunnel: [w647] -> w645
                    tunnel: w646 -> [w653]
                    tunnel: w645 -> [w652]
                    frame #0 {
                      w647 = 0.84 ("target_ir_l")
                      w648 = 0.84 ("target_ir_r")
                      n277 = call "integal_caribat_squence.vi"("inner_b_ir"=0.4, "inner_f_ir"=0.8, "target_ir_l"=w647, "target_ir_r"=w648, "precision"=0.008) -> ()
                    }
                    frame #1 {
                      n278 = call "integal_pickup_sequence .vi"("store_pos"=u8 156, "pick_pos"=u8 52, "target_ir_l"=w652, "target_ir_r"=w653, "precision"=0.04) -> ()
                    }
                  }
                }
                frame #4 {
                  n279 = flat-sequence {
                    frame #0 {
                      n280 = call "turn_.vi"("delay"=u32 3000, "Carzeta"=180.0) -> ()  [unwired: 10 in]
                    }
                    frame #1 {
                      n281 = expression code="x*115"(5.0) -> (w662:dbl)
                      n282 = call "move_.vi"("Enum"=enum16{"hold", "f", "b"}."f", "delay"=u32 6000, "D"=w662) -> ()  [unwired: 1 in]
                    }
                  }
                }
                frame #5 {
                  n283 = flat-sequence {
                    frame #0 {
                      n284 = call "turn_.vi"("delay"=u32 3000, "Carzeta"=-90.0) -> ()  [unwired: 10 in]
                    }
                    frame #1 {
                      n285 = expression code="x*115"(1.0) -> (w668:dbl)
                      n286 = call "move_.vi"("Enum"=enum16{"hold", "f", "b"}."f", "delay"=u32 1500, "D"=w668) -> ()  [unwired: 1 in]
                    }
                  }
                }
              }
            }
            frame 5 {
              n287 = stacked-sequence {
                frame #0 {
                  # "move up"
                  n288 = flat-sequence {
                    frame #0 {
                      n289 = call "turn_.vi"("delay"=u32 3500, "Carzeta"=135.0) -> ()  [unwired: 10 in]
                    }
                    frame #1 {
                      n290 = expression code="x*115"(4.4) -> (w671:dbl)
                      n291 = call "move_.vi"("Enum"=enum16{"hold", "f", "b"}."f", "delay"=u32 5000, "D"=w671) -> ()  [unwired: 1 in]
                    }
                  }
                }
                frame #1 {
                  # "move left"
                  n292 = flat-sequence {
                    frame #0 {
                      n293 = call "turn_.vi"("delay"=u32 3500, "Carzeta"=90.0) -> ()  [unwired: 10 in]
                    }
                    frame #1 {
                      n294 = expression code="x*115"(4.0) -> (w679:dbl)
                      n295 = call "move_.vi"("Enum"=enum16{"hold", "f", "b"}."f", "delay"=u32 4500, "D"=w679) -> ()  [unwired: 1 in]
                    }
                  }
                }
                frame #2 {
                  # "take green block"
                  n296 = flat-sequence {
                    tunnel: [w684] -> w682
                    tunnel: [w683] -> w681
                    tunnel: w682 -> [w689]
                    tunnel: w681 -> [w688]
                    frame #0 {
                      w683 = 0.84 ("target_ir_l")
                      w684 = 0.84 ("target_ir_r")
                      n297 = call "integal_caribat_squence.vi"("inner_b_ir"=0.4, "inner_f_ir"=0.8, "target_ir_l"=w683, "target_ir_r"=w684, "precision"=0.008) -> ()
                    }
                    frame #1 {
                      n298 = call "integal_pickup_sequence .vi"("store_pos"=u8 154, "pick_pos"=u8 52, "target_ir_l"=w688, "target_ir_r"=w689, "precision"=0.05) -> ()
                    }
                  }
                }
                frame #3 {
                  # "move down"
                  n299 = flat-sequence {
                    frame #0 {
                      n300 = call "turn_.vi"("delay"=u32 2500, "Carzeta"=90.0) -> ()  [unwired: 10 in]
                    }
                    frame #1 {
                      n301 = expression code="x*115"(9.0) -> (w696:dbl)
                      n302 = call "move_v2.vi"("delay"=u32 2500, "Enum"=enum16{"hold", "f", "b"}."f", "D"=w696) -> ()  [unwired: 1 in]
                    }
                  }
                }
                frame #4 {
                  # "move right"
                  n303 = flat-sequence {
                    frame #0 {
                      n304 = call "turn_.vi"("delay"=u32 2500, "Carzeta"=90.0) -> ()  [unwired: 10 in]
                    }
                    frame #1 {
                      n305 = expression code="x*115"(8.0) -> (w702:dbl)
                      n306 = call "move_v2.vi"("delay"=u32 2500, "Enum"=enum16{"hold", "f", "b"}."f", "D"=w702) -> ()  [unwired: 1 in]
                    }
                  }
                }
                frame #5 {
                  # "take red block"
                  n307 = flat-sequence {
                    tunnel: [w708] -> w706
                    tunnel: [w707] -> w705
                    tunnel: w706 -> [w713]
                    tunnel: w705 -> [w712]
                    frame #0 {
                      w707 = 0.84 ("target_ir_l")
                      w708 = 0.84 ("target_ir_r")
                      n308 = call "integal_caribat_squence.vi"("inner_b_ir"=0.4, "inner_f_ir"=0.8, "target_ir_l"=w707, "target_ir_r"=w708, "precision"=0.008) -> ()
                    }
                    frame #1 {
                      n309 = call "integal_pickup_sequence .vi"("store_pos"=u8 183, "pick_pos"=u8 52, "target_ir_l"=w712, "target_ir_r"=w713, "precision"=0.05) -> ()
                    }
                  }
                }
                frame #6 {
                  # "drop green"
                  n310 = call "integal_return.vi"("servo 3 dropfront"=u8 52, "servo 3 pickBack"=u8 153) -> ()
                }
                frame #7 {
                  n311 = flat-sequence {
                    frame #0 {
                      n312 = call "move_.vi"("Enum"=enum16{"hold", "f", "b"}."b", "delay"=u32 1500, "D"=115.0) -> ()  [unwired: 1 in]
                    }
                    frame #1 {
                      n313 = call "turn_.vi"("delay"=u32 2500, "Carzeta"=-90.0) -> ()  [unwired: 10 in]
                    }
                  }
                }
                frame #8 {
                  # "take yellow"
                  n314 = flat-sequence {
                    tunnel: [w727] -> w725
                    tunnel: [w726] -> w724
                    tunnel: w725 -> [w732]
                    tunnel: w724 -> [w731]
                    frame #0 {
                      w726 = 0.85 ("target_ir_l")
                      w727 = 0.85 ("target_ir_r")
                      n315 = call "integal_caribat_squence.vi"("inner_b_ir"=0.4, "inner_f_ir"=0.8, "target_ir_l"=w726, "target_ir_r"=w727, "precision"=0.01) -> ()
                    }
                    frame #1 {
                      n316 = call "integal_pickup_sequence .vi"("store_pos"=u8 154, "pick_pos"=u8 53, "target_ir_l"=w731, "target_ir_r"=w732, "precision"=0.05) -> ()
                    }
                  }
                }
                frame #9 {
                  n317 = flat-sequence {
                    frame #0 {
                      n318 = call "turn_.vi"("delay"=u32 2500, "Carzeta"=-90.0) -> ()  [unwired: 10 in]
                    }
                    frame #1 {
                      n319 = expression code="x*115"(7.0) -> (w739:dbl)
                      n320 = call "move_v2.vi"("delay"=u32 2000, "Enum"=enum16{"hold", "f", "b"}."f", "D"=w739) -> ()  [unwired: 1 in]
                    }
                  }
                }
                frame #10 {
                  n321 = flat-sequence {
                    frame #0 {
                      n322 = call "turn_.vi"("delay"=u32 2500, "Carzeta"=-91.0) -> ()  [unwired: 10 in]
                    }
                    frame #1 {
                      n323 = expression code="x*115"(9.0) -> (w745:dbl)
                      n324 = call "move_v2.vi"("delay"=u32 2000, "Enum"=enum16{"hold", "f", "b"}."f", "D"=w745) -> ()  [unwired: 1 in]
                    }
                  }
                }
                frame #11 {
                  n325 = flat-sequence {
                    tunnel: [w757] -> w749
                    tunnel: w749 -> [w759]
                    tunnel: [w759] -> w748
                    tunnel: w748 -> [w761]
                    frame #0 {
                      n326 = call "turn_.vi"("delay"=u32 2500, "Carzeta"=90.0) -> ()  [unwired: 10 in]
                    }
                    frame #1 {
                      n327 = call "integal_caribat_squence.vi"("inner_b_ir"=0.4, "inner_f_ir"=0.8, "target_ir_l"=0.84, "target_ir_r"=0.84, "precision"=0.01) -> ()
                    }
                    frame #2 {
                      w757 = u8 52 ("servo 3 dropfront")
                      n328 = call "integal_return.vi"("servo 3 dropfront"=w757, "servo 3 pickBack"=u8 153) -> ()
                    }
                    frame #3 {
                      n329 = call "servo_pickfromback_sequence.vi"("pick_pos"=u8 182 ("servo 3")) -> ()
                    }
                    frame #4 {
                      n330 = global write "GlobalVar.vi" "servo 3"(w761) -> ()
                    }
                  }
                }
                frame #12 {
                  n331 = flat-sequence {
                    frame #0 {
                      n332 = call "turn_.vi"("delay"=u32 2500, "Carzeta"=90.0) -> ()  [unwired: 10 in]
                    }
                    frame #1 {
                      n333 = expression code="x*115"(4.5) -> (w766:dbl)
                      n334 = call "move_.vi"("Enum"=enum16{"hold", "f", "b"}."f", "delay"=u32 5000, "D"=w766) -> ()  [unwired: 1 in]
                    }
                  }
                }
                frame #13 {
                  n335 = flat-sequence {
                    frame #0 {
                      n336 = call "turn_.vi"("delay"=u32 2500, "Carzeta"=90.0) -> ()  [unwired: 10 in]
                    }
                    frame #1 {
                      n337 = expression code="x*115"(4.3) -> (w772:dbl)
                      n338 = call "move_.vi"("Enum"=enum16{"hold", "f", "b"}."f", "delay"=u32 4500, "D"=w772) -> ()  [unwired: 1 in]
                    }
                  }
                }
              }
            }
            frame 6 {
              n339 = stacked-sequence {
                frame #0 {
                  n340 = flat-sequence {
                    tunnel: [w778] -> w776
                    tunnel: [w777] -> w774
                    tunnel: w776 -> [w785]
                    tunnel: [w784] -> w775
                    tunnel: w774 -> [w784]
                    tunnel: w775 -> [w788]
                    frame #0 {
                      n341 = call "turn_offset.vi"("x2"=5.0, "x1"=7.0, "y2"=11.0, "y1"=12.0) -> ("dis_"=w777:dbl, "zeta"=w778:dbl)
                    }
                    frame #1 {
                      n342 = expression code="45+x"(w785) -> (w783:dbl)
                      n343 = call "turn_.vi"("delay"=u32 5000, "Carzeta"=w783) -> ()  [unwired: 10 in]
                    }
                    frame #2 {
                      n344 = Subtract(x=115.0, y=w788) -> (x-y=w787:dbl)
                      n345 = call "move_.vi"("Enum"=enum16{"hold", "f", "b"}."b", "delay"=u32 2000, "D"=w787) -> ()  [unwired: 1 in]
                    }
                  }
                }
                frame #1 {
                  n346 = flat-sequence {
                    frame #0 {
                      n347 = call "turn_.vi"("delay"=u32 3500, "Carzeta"=90.0) -> ()  [unwired: 10 in]
                    }
                    frame #1 {
                      n348 = expression code="x*115"(4.5) -> (w796:dbl)
                      n349 = call "move_.vi"("Enum"=enum16{"hold", "f", "b"}."f", "delay"=u32 5000, "D"=w796) -> ()  [unwired: 1 in]
                    }
                  }
                }
                frame #2 {
                  n350 = flat-sequence {
                    tunnel: [w801] -> w799
                    tunnel: [w800] -> w798
                    tunnel: w799 -> [w806]
                    tunnel: w798 -> [w805]
                    frame #0 {
                      w800 = 0.84 ("target_ir_l")
                      w801 = 0.84 ("target_ir_r")
                      n351 = call "integal_caribat_squence.vi"("inner_b_ir"=0.4, "inner_f_ir"=0.8, "target_ir_l"=w800, "target_ir_r"=w801, "precision"=0.008) -> ()
                    }
                    frame #1 {
                      n352 = call "integal_pickup_sequence .vi"("store_pos"=u8 156, "pick_pos"=u8 51, "target_ir_l"=w805, "target_ir_r"=w806, "precision"=0.05) -> ()
                    }
                  }
                }
                frame #3 {
                  n353 = flat-sequence {
                    frame #0 {
                      n354 = call "turn_.vi"("delay"=u32 5000, "Carzeta"=179.0) -> ()  [unwired: 10 in]
                    }
                    frame #1 {
                      n355 = expression code="x*115"(7.0) -> (w813:dbl)
                      n356 = call "move_v2.vi"("delay"=u32 2000, "Enum"=enum16{"hold", "f", "b"}."f", "D"=w813) -> ()  [unwired: 1 in]
                    }
                  }
                }
                frame #4 {
                  n357 = flat-sequence {
                    frame #0 {
                      n358 = call "turn_.vi"("delay"=u32 3000, "Carzeta"=-90.0) -> ()  [unwired: 10 in]
                    }
                    frame #1 {
                      n359 = expression code="x*115"(6.0) -> (w820:dbl)
                      n360 = call "move_.vi"("Enum"=enum16{"hold", "f", "b"}."f", "delay"=u32 6500, "D"=w820) -> ()  [unwired: 1 in]
                    }
                  }
                }
                frame #5 {
                  n361 = flat-sequence {
                    tunnel: [w825] -> w823
                    tunnel: [w824] -> w822
                    tunnel: w823 -> [w830]
                    tunnel: w822 -> [w829]
                    frame #0 {
                      w824 = 0.84 ("target_ir_l")
                      w825 = 0.84 ("target_ir_r")
                      n362 = call "integal_caribat_squence.vi"("inner_b_ir"=0.4, "inner_f_ir"=0.8, "target_ir_l"=w824, "target_ir_r"=w825, "precision"=0.008) -> ()
                    }
                    frame #1 {
                      n363 = call "integal_pickup_sequence .vi"("store_pos"=u8 183, "pick_pos"=u8 52, "target_ir_l"=w829, "target_ir_r"=w830, "precision"=0.05) -> ()
                    }
                  }
                }
                frame #6 {
                  # "154"
                  n364 = call "integal_return.vi"("servo 3 dropfront"=u8 52, "servo 3 pickBack"=u8 155) -> ()
                }
                frame #7 {
                  n365 = flat-sequence {
                    frame #0 {
                      n366 = expression code="x*115"(1.0) -> (w839:dbl)
                      n367 = call "move_.vi"("Enum"=enum16{"hold", "f", "b"}."b", "delay"=u32 1500, "D"=w839) -> ()  [unwired: 1 in]
                    }
                    frame #1 {
                      n368 = call "turn_.vi"("delay"=u32 3000, "Carzeta"=90.0) -> ()  [unwired: 10 in]
                    }
                    frame #2 {
                      n369 = expression code="x*115"(3.0) -> (w845:dbl)
                      n370 = call "move_.vi"("Enum"=enum16{"hold", "f", "b"}."f", "delay"=u32 3500, "D"=w845) -> ()  [unwired: 1 in]
                    }
                    frame #3 {
                      n371 = call "turn_.vi"("delay"=u32 3000, "Carzeta"=-90.0) -> ()  [unwired: 10 in]
                    }
                  }
                }
                frame #8 {
                  n372 = flat-sequence {
                    frame #0 {
                      n373 = call "integal_caribat_squence.vi"("inner_b_ir"=0.4, "inner_f_ir"=0.8, "target_ir_l"=0.84, "target_ir_r"=0.84, "precision"=0.008) -> ()
                    }
                    frame #1 {
                      n374 = call "servo_pickup_sequence.vi"("servo 3"=u8 53) -> ()
                    }
                  }
                }
                frame #9 {
                  n375 = flat-sequence {
                    frame #0 {
                      n376 = call "turn_.vi"("delay"=u32 3000, "Carzeta"=-90.0) -> ()  [unwired: 10 in]
                    }
                    frame #1 {
                      n377 = expression code="x*115"(10.0) -> (w857:dbl)
                      n378 = call "move_v2.vi"("delay"=u32 2000, "Enum"=enum16{"hold", "f", "b"}."f", "D"=w857) -> ()  [unwired: 1 in]
                    }
                  }
                }
                frame #10 {
                  n379 = flat-sequence {
                    frame #0 {
                      n380 = call "turn_.vi"("delay"=u32 3000, "Carzeta"=-90.0) -> ()  [unwired: 10 in]
                    }
                    frame #1 {
                      n381 = expression code="x*115"(5.0) -> (w864:dbl)
                      n382 = call "move_.vi"("Enum"=enum16{"hold", "f", "b"}."f", "delay"=u32 5500, "D"=w864) -> ()  [unwired: 1 in]
                    }
                  }
                }
                frame #11 {
                  n383 = flat-sequence {
                    frame #0 {
                      n384 = call "turn_.vi"("delay"=u32 3000, "Carzeta"=90.0) -> ()  [unwired: 10 in]
                    }
                    frame #1 {
                      n385 = call "integal_caribat_squence.vi"("inner_b_ir"=0.4, "inner_f_ir"=0.8, "target_ir_l"=0.84, "target_ir_r"=0.84, "precision"=0.008) -> ()
                    }
                    frame #2 {
                      n386 = call "servo_return_block_sequence.vi"("servo 3"=u8 52) -> ()
                    }
                  }
                }
                frame #12 {
                  # "keep red 2 home"
                  n387 = flat-sequence {
                    frame #0 {
                      n388 = call "servo_pickfromback_sequence.vi"("pick_pos"=u8 182) -> ()
                    }
                    frame #1 {
                      n389 = global write "GlobalVar.vi" "servo 3"(u8 52 ("servo 3")) -> ()
                    }
                  }
                  n390 = flat-sequence {
                    frame #0 {
                      n391 = call "turn_.vi"("delay"=u32 5000, "Carzeta"=180.0) -> ()  [unwired: 10 in]
                    }
                    frame #1 {
                      n392 = expression code="x*115"(5.0) -> (w880:dbl)
                      n393 = call "move_.vi"("Enum"=enum16{"hold", "f", "b"}."f", "delay"=u32 7000, "D"=w880) -> ()  [unwired: 1 in]
                    }
                  }
                }
                frame #13 {
                  # "turn 2 parking"
                  n394 = flat-sequence {
                    frame #0 {
                      n395 = call "turn_.vi"("delay"=u32 2500, "Carzeta"=71.0) -> ()  [unwired: 10 in]
                    }
                    frame #1 {
                      n396 = expression code="x*115"(2.0) -> (w886:dbl)
                      n397 = call "move_.vi"("Enum"=enum16{"hold", "f", "b"}."f", "delay"=u32 2500, "D"=w886) -> ()  [unwired: 1 in]
                    }
                  }
                }
              }
            }
            frame 7 {
            }
            frame 8 {
              n398 = stacked-sequence {
                frame #0 {
                  n399 = flat-sequence {
                    tunnel: [w892] -> w890
                    tunnel: [w891] -> w888
                    tunnel: w890 -> [w899]
                    tunnel: [w898] -> w889
                    tunnel: w888 -> [w898]
                    tunnel: w889 -> [w901]
                    frame #0 {
                      n400 = call "turn_offset.vi"("x2"=18.0, "x1"=15.0, "y2"=10.0, "y1"=9.0) -> ("dis_"=w891:dbl, "zeta"=w892:dbl)
                    }
                    frame #1 {
                      n401 = expression code="45+x"(w899) -> (w897:dbl)
                      n402 = call "turn_.vi"("delay"=u32 3000, "Carzeta"=w897) -> ()  [unwired: 10 in]
                    }
                    frame #2 {
                      n403 = call "move_.vi"("Enum"=enum16{"hold", "f", "b"}."b", "delay"=u32 2000, "D"=w901) -> ()  [unwired: 1 in]
                    }
                  }
                }
                frame #1 {
                  n404 = flat-sequence {
                    frame #0 {
                      n405 = call "turn_.vi"("delay"=u32 3000, "Carzeta"=90.0) -> ()  [unwired: 10 in]
                    }
                    frame #1 {
                      n406 = expression code="x*115"(3.5) -> (w908:dbl)
                      n407 = call "move_.vi"("Enum"=enum16{"hold", "f", "b"}."f", "delay"=u32 4500, "D"=w908) -> ()  [unwired: 1 in]
                    }
                  }
                }
                frame #2 {
                  n408 = flat-sequence {
                    frame #0 {
                      n409 = call "turn_.vi"("delay"=u32 3500, "Carzeta"=-90.0) -> ()  [unwired: 10 in]
                    }
                    frame #1 {
                      n410 = expression code="x*115"(3.0) -> (w914:dbl)
                      n411 = call "move_.vi"("Enum"=enum16{"hold", "f", "b"}."f", "delay"=u32 3500, "D"=w914) -> ()  [unwired: 1 in]
                    }
                    frame #2 {
                      n412 = call "turn_.vi"("delay"=u32 3500, "Carzeta"=90.0) -> ()  [unwired: 10 in]
                    }
                  }
                }
                frame #3 {
                  n413 = flat-sequence {
                    tunnel: [w921] -> w919
                    tunnel: [w920] -> w918
                    tunnel: w919 -> [w926]
                    tunnel: w918 -> [w925]
                    frame #0 {
                      w920 = 0.84 ("target_ir_l")
                      w921 = 0.84 ("target_ir_r")
                      n414 = call "integal_caribat_squence.vi"("inner_b_ir"=0.4, "inner_f_ir"=0.8, "target_ir_l"=w920, "target_ir_r"=w921, "precision"=0.008) -> ()
                    }
                    frame #1 {
                      n415 = call "integal_pickup_sequence .vi"("store_pos"=u8 156, "pick_pos"=u8 52, "target_ir_l"=w925, "target_ir_r"=w926, "precision"=0.05) -> ()
                    }
                  }
                }
                frame #4 {
                  n416 = flat-sequence {
                    frame #0 {
                      n417 = call "turn_.vi"("delay"=u32 3000, "Carzeta"=90.0) -> ()  [unwired: 10 in]
                    }
                    frame #1 {
                      n418 = expression code="x*115"(4.0) -> (w934:dbl)
                      n419 = call "move_.vi"("Enum"=enum16{"hold", "f", "b"}."f", "delay"=u32 4500, "D"=w934) -> ()  [unwired: 1 in]
                    }
                  }
                }
                frame #5 {
                  n420 = flat-sequence {
                    frame #0 {
                      n421 = call "turn_.vi"("delay"=u32 3000, "Carzeta"=90.0) -> ()  [unwired: 10 in]
                    }
                    frame #1 {
                      n422 = expression code="x*115"(10.0) -> (w939:dbl)
                      n423 = call "move_v2.vi"("delay"=u32 3000, "Enum"=enum16{"hold", "f", "b"}."f", "D"=w939) -> ()  [unwired: 1 in]
                    }
                  }
                }
                frame #6 {
                  n424 = flat-sequence {
                    frame #0 {
                      n425 = call "turn_.vi"("delay"=u32 3000, "Carzeta"=90.0) -> ()  [unwired: 10 in]
                    }
                    frame #1 {
                      n426 = expression code="x*115"(4.0) -> (w946:dbl)
                      n427 = call "move_.vi"("Enum"=enum16{"hold", "f", "b"}."f", "delay"=u32 4500, "D"=w946) -> ()  [unwired: 1 in]
                    }
                  }
                }
                frame #7 {
                  n428 = flat-sequence {
                    tunnel: [w951] -> w949
                    tunnel: [w950] -> w948
                    tunnel: w949 -> [w956]
                    tunnel: w948 -> [w955]
                    frame #0 {
                      w950 = 0.84 ("target_ir_l")
                      w951 = 0.84 ("target_ir_r")
                      n429 = call "integal_caribat_squence.vi"("inner_b_ir"=0.4, "inner_f_ir"=0.8, "target_ir_l"=w950, "target_ir_r"=w951, "precision"=0.008) -> ()
                    }
                    frame #1 {
                      n430 = call "integal_pickup_sequence .vi"("store_pos"=u8 183, "pick_pos"=u8 52, "target_ir_l"=w955, "target_ir_r"=w956, "precision"=0.04) -> ()
                    }
                  }
                }
                frame #8 {
                  # "154"
                  n431 = call "integal_return.vi"("servo 3 dropfront"=u8 52, "servo 3 pickBack"=u8 154) -> ()
                }
                frame #9 {
                  n432 = flat-sequence {
                    frame #0 {
                      n433 = expression code="x*115"(2.0) -> (w964:dbl)
                      n434 = call "move_.vi"("Enum"=enum16{"hold", "f", "b"}."b", "delay"=u32 2500, "D"=w964) -> ()  [unwired: 1 in]
                    }
                    frame #1 {
                      n435 = call "turn_.vi"("delay"=u32 3000, "Carzeta"=-90.0) -> ()  [unwired: 10 in]
                    }
                  }
                }
                frame #10 {
                  n436 = flat-sequence {
                    frame #0 {
                      n437 = call "integal_caribat_squence.vi"("inner_b_ir"=0.4, "inner_f_ir"=0.8, "target_ir_l"=0.84, "target_ir_r"=0.84, "precision"=0.008) -> ()
                    }
                    frame #1 {
                      n438 = call "servo_pickup_sequence.vi"("servo 3"=u8 52) -> ()
                    }
                  }
                }
                frame #11 {
                  n439 = flat-sequence {
                    frame #0 {
                      n440 = call "turn_.vi"("delay"=u32 5000, "Carzeta"=-168.69) -> ()  [unwired: 10 in]
                    }
                    frame #1 {
                      n441 = expression code="x*115"(10.19) -> (w977:dbl)
                      n442 = call "move_v2.vi"("delay"=u32 2500, "Enum"=enum16{"hold", "f", "b"}."f", "D"=w977) -> ()  [unwired: 1 in]
                    }
                    frame #2 {
                      n443 = call "turn_.vi"("delay"=u32 3500, "Carzeta"=-102.0) -> ()  [unwired: 10 in]
                    }
                    frame #3 {
                      n444 = expression code="x*115"(4.5) -> (w984:dbl)
                      n445 = call "move_.vi"("Enum"=enum16{"hold", "f", "b"}."f", "delay"=u32 4500, "D"=w984) -> ()  [unwired: 1 in]
                    }
                    frame #4 {
                      n446 = call "turn_.vi"("delay"=u32 3000, "Carzeta"=90.0) -> ()  [unwired: 10 in]
                    }
                  }
                }
                frame #12 {
                  n447 = flat-sequence {
                    frame #0 {
                      n448 = call "integal_caribat_squence.vi"("inner_b_ir"=0.4, "inner_f_ir"=0.8, "target_ir_l"=0.84, "target_ir_r"=0.84, "precision"=0.008) -> ()
                    }
                    frame #1 {
                      n449 = call "servo_return_block_sequence.vi"("servo 3"=u8 52) -> ()
                    }
                  }
                }
                frame #13 {
                  n450 = flat-sequence {
                    frame #0 {
                      n451 = call "servo_pickfromback_sequence.vi"("pick_pos"=u8 182) -> ()
                    }
                    frame #1 {
                      n452 = global write "GlobalVar.vi" "servo 3"(u8 100 ("servo 3")) -> ()
                    }
                  }
                  n453 = flat-sequence {
                    tunnel: w994 -> [w1013]
                    frame #0 {
                      n454 = call "turn_.vi"("delay"=u32 3000, "Carzeta"=90.0) -> ()  [unwired: 10 in]
                    }
                    frame #1 {
                      n455 = expression code="x*115"(1.5) -> (w1005:dbl)
                      n456 = call "move_.vi"("Enum"=enum16{"hold", "f", "b"}."f", "delay"=u32 2300, "D"=w1005) -> ()  [unwired: 1 in]
                    }
                    frame #2 {
                      n457 = call "turn_.vi"("delay"=u32 3000, "Carzeta"=90.0) -> ()  [unwired: 10 in]
                    }
                    frame #3 {
                      n458 = expression code="x*115"(3.5) -> (w1011:dbl)
                      n459 = call "move_.vi"("Enum"=enum16{"hold", "f", "b"}."f", "delay"=u32 2300, "D"=w1011) -> ()  [unwired: 1 in]
                    }
                    frame #4 {
                      n460 = call "turn_.vi"("delay"=u32 3000, "Carzeta"=w1013) -> ()  [unwired: 10 in]
                    }
                    frame #5 {
                    }
                  }
                  n461 = call "turn_offset.vi"("x2"=18.0, "x1"=15.0, "y2"=10.0, "y1"=9.0) -> ("zeta"=w994:dbl)  [unwired: 1 out]
                }
              }
            }
            frame 9 {
              n462 = stacked-sequence {
                frame #0 {
                  n463 = flat-sequence {
                    frame #0 {
                      n464 = expression code="x-45"(18.435 ("zeta")) -> (w1016:dbl)
                      n465 = call "turn_.vi"("delay"=u32 3000, "Carzeta"=w1016) -> ()  [unwired: 10 in]
                    }
                    frame #1 {
                      n466 = call "move_.vi"("Enum"=enum16{"hold", "f", "b"}."f", "delay"=u32 2000, "D"=50.0) -> ()  [unwired: 1 in]
                    }
                  }
                }
                frame #1 {
                  n467 = flat-sequence {
                    frame #0 {
                      n468 = call "turn_.vi"("delay"=u32 2000, "Carzeta"=-38.66) -> ()  [unwired: 10 in]
                    }
                    frame #1 {
                      n469 = expression code="x*115"(6.8) -> (w1024:dbl)
                      n470 = call "move_v2.vi"("delay"=u32 2000, "Enum"=enum16{"hold", "f", "b"}."f", "D"=w1024) -> ()  [unwired: 1 in]
                    }
                    frame #2 {
                      n471 = call "turn_.vi"("delay"=u32 2000, "Carzeta"=-51.34) -> ()  [unwired: 10 in]
                    }
                  }
                }
                frame #2 {
                  n472 = flat-sequence {
                    tunnel: [w1032] -> w1030
                    tunnel: [w1031] -> w1029
                    tunnel: w1030 -> [w1037]
                    tunnel: w1029 -> [w1036]
                    frame #0 {
                      w1031 = 0.84 ("target_ir_l")
                      w1032 = 0.84 ("target_ir_r")
                      n473 = call "integal_caribat_squence.vi"("inner_b_ir"=0.4, "inner_f_ir"=0.8, "target_ir_l"=w1031, "target_ir_r"=w1032, "precision"=0.008) -> ()
                    }
                    frame #1 {
                      n474 = call "integal_pickup_sequence .vi"("store_pos"=u8 183, "pick_pos"=u8 52, "target_ir_l"=w1036, "target_ir_r"=w1037, "precision"=0.04) -> ()
                    }
                  }
                }
                frame #3 {
                  n475 = flat-sequence {
                    frame #0 {
                      n476 = call "turn_.vi"("delay"=u32 5000, "Carzeta"=187.125) -> ()  [unwired: 10 in]
                    }
                    frame #1 {
                      n477 = expression code="x*115"(8.06) -> (w1044:dbl)
                      n478 = call "move_v2.vi"("delay"=u32 2500, "Enum"=enum16{"hold", "f", "b"}."f", "D"=w1044) -> ()  [unwired: 1 in]
                    }
                    frame #2 {
                      n479 = call "turn_.vi"("delay"=u32 700, "Carzeta"=-7.13) -> ()  [unwired: 10 in]
                    }
                  }
                }
                frame #4 {
                  n480 = flat-sequence {
                    tunnel: [w1052] -> w1050
                    tunnel: [w1051] -> w1049
                    tunnel: w1050 -> [w1057]
                    tunnel: w1049 -> [w1056]
                    frame #0 {
                      w1051 = 0.84 ("target_ir_l")
                      w1052 = 0.84 ("target_ir_r")
                      n481 = call "integal_caribat_squence.vi"("inner_b_ir"=0.4, "inner_f_ir"=0.8, "target_ir_l"=w1051, "target_ir_r"=w1052, "precision"=0.008) -> ()
                    }
                    frame #1 {
                      n482 = call "integal_pickup_sequence .vi"("store_pos"=u8 155, "pick_pos"=u8 52, "target_ir_l"=w1056, "target_ir_r"=w1057, "precision"=0.04) -> ()
                    }
                  }
                }
                frame #5 {
                  # "154"
                  n483 = call "integal_return.vi"("servo 3 dropfront"=u8 52, "servo 3 pickBack"=u8 183) -> ()
                }
                frame #6 {
                  n484 = flat-sequence {
                    frame #0 {
                      n485 = expression code="x*115"(2.0 ("zeta")) -> (w1063:dbl)
                      n486 = call "move_.vi"("Enum"=enum16{"hold", "f", "b"}."b", "delay"=u32 2500, "D"=w1063) -> ()  [unwired: 1 in]
                    }
                    frame #1 {
                      n487 = call "turn_.vi"("delay"=u32 3000, "Carzeta"=-90.0 ("zeta")) -> ()  [unwired: 10 in]
                    }
                    frame #2 {
                      n488 = expression code="x*115"(2.0 ("zeta")) -> (w1069:dbl)
                      n489 = call "move_.vi"("Enum"=enum16{"hold", "f", "b"}."f", "delay"=u32 2500, "D"=w1069) -> ()  [unwired: 1 in]
                    }
                  }
                }
                frame #7 {
                  n490 = flat-sequence {
                    tunnel: [w1076] -> w1074
                    tunnel: [w1075] -> w1073
                    tunnel: w1074 -> [w1081]
                    tunnel: w1073 -> [w1080]
                    frame #0 {
                      w1075 = 0.84 ("target_ir_l")
                      w1076 = 0.84 ("target_ir_r")
                      n491 = call "integal_caribat_squence.vi"("inner_b_ir"=0.4, "inner_f_ir"=0.8, "target_ir_l"=w1075, "target_ir_r"=w1076, "precision"=0.008) -> ()
                    }
                    frame #1 {
                      n492 = call "integal_pickup_sequence .vi"("store_pos"=u8 183, "pick_pos"=u8 52, "target_ir_l"=w1080, "target_ir_r"=w1081, "precision"=0.04) -> ()
                    }
                  }
                }
                frame #8 {
                  # "154"
                  n493 = call "integal_return.vi"("servo 3 dropfront"=u8 52, "servo 3 pickBack"=u8 154) -> ()
                }
                frame #9 {
                  n494 = flat-sequence {
                    frame #0 {
                      n495 = call "turn_.vi"("delay"=u32 3000, "Carzeta"=-90.0 ("zeta")) -> ()  [unwired: 10 in]
                    }
                    frame #1 {
                      n496 = expression code="x*115"(2.0 ("zeta")) -> (w1094:dbl)
                      n497 = call "move_.vi"("Enum"=enum16{"hold", "f", "b"}."f", "delay"=u32 2500, "D"=w1094) -> ()  [unwired: 1 in]
                    }
                    frame #2 {
                      n498 = call "turn_.vi"("delay"=u32 3000, "Carzeta"=-90.0 ("zeta")) -> ()  [unwired: 10 in]
                    }
                    frame #3 {
                      n499 = expression code="x*115"(7.5 ("zeta")) -> (w1100:dbl)
                      n500 = call "move_.vi"("Enum"=enum16{"hold", "f", "b"}."f", "delay"=u32 8500, "D"=w1100) -> ()  [unwired: 1 in]
                    }
                    frame #4 {
                      n501 = call "turn_.vi"("delay"=u32 3000, "Carzeta"=-110.0 ("zeta")) -> ()  [unwired: 10 in]
                    }
                    frame #5 {
                      n502 = expression code="x*115"(2.5 ("zeta")) -> (w1103:dbl)
                      n503 = call "move_.vi"("Enum"=enum16{"hold", "f", "b"}."f", "delay"=u32 6500, "D"=w1103) -> ()  [unwired: 1 in]
                    }
                  }
                  n504 = flat-sequence {
                    frame #0 {
                      n505 = call "servo_pickfromback_sequence.vi"("pick_pos"=u8 182) -> ()
                    }
                    frame #1 {
                      n506 = global write "GlobalVar.vi" "servo 3"(u8 100 ("servo 3")) -> ()
                    }
                  }
                }
              }
            }
            frame 10 {
              n507 = stacked-sequence {
                frame #0 {
                  n508 = flat-sequence {
                    frame #0 {
                      n509 = expression code="45-x"(18.43 ("zeta")) -> (w1108:dbl)
                      n510 = call "turn_.vi"("delay"=u32 3000, "Carzeta"=w1108) -> ()  [unwired: 10 in]
                    }
                    frame #1 {
                      n511 = call "move_.vi"("Enum"=enum16{"hold", "f", "b"}."b", "delay"=u32 2000, "D"=50.0) -> ()  [unwired: 1 in]
                    }
                  }
                }
                frame #1 {
                  n512 = flat-sequence {
                    frame #0 {
                      n513 = call "turn_.vi"("delay"=u32 5000, "Carzeta"=-263.66) -> ()  [unwired: 10 in]
                    }
                    frame #1 {
                      n514 = expression code="x*115"(6.7) -> (w1116:dbl)
                      n515 = call "move_v2.vi"("delay"=u32 3000, "Enum"=enum16{"hold", "f", "b"}."f", "D"=w1116) -> ()  [unwired: 1 in]
                    }
                    frame #2 {
                      n516 = call "turn_.vi"("delay"=u32 2000, "Carzeta"=51.34) -> ()  [unwired: 10 in]
                    }
                  }
                }
                frame #2 {
                  n517 = flat-sequence {
                    frame #0 {
                      n518 = call "turn_.vi"("delay"=u32 3000, "Carzeta"=90.0 ("zeta")) -> ()  [unwired: 10 in]
                    }
                    frame #1 {
                      n519 = expression code="x*115"(2.0 ("zeta")) -> (w1126:dbl)
                      n520 = call "move_.vi"("Enum"=enum16{"hold", "f", "b"}."f", "delay"=u32 2500, "D"=w1126) -> ()  [unwired: 1 in]
                    }
                    frame #2 {
                      n521 = call "turn_.vi"("delay"=u32 3000, "Carzeta"=90.0 ("zeta")) -> ()  [unwired: 10 in]
                    }
                    frame #3 {
                      n522 = expression code="x*115"(7.0 ("zeta")) -> (w1129:dbl)
                      n523 = call "move_.vi"("Enum"=enum16{"hold", "f", "b"}."f", "delay"=u32 6500, "D"=w1129) -> ()  [unwired: 1 in]
                    }
                  }
                }
                frame #3 {
                  n524 = flat-sequence {
                    tunnel: [w1136] -> w1134
                    tunnel: [w1135] -> w1133
                    tunnel: w1134 -> [w1141]
                    tunnel: w1133 -> [w1140]
                    frame #0 {
                      w1135 = 0.84 ("target_ir_l")
                      w1136 = 0.84 ("target_ir_r")
                      n525 = call "integal_caribat_squence.vi"("inner_b_ir"=0.4, "inner_f_ir"=0.8, "target_ir_l"=w1135, "target_ir_r"=w1136, "precision"=0.008) -> ()
                    }
                    frame #1 {
                      n526 = call "integal_pickup_sequence .vi"("store_pos"=u8 154, "pick_pos"=u8 52, "target_ir_l"=w1140, "target_ir_r"=w1141, "precision"=0.04) -> ()
                    }
                  }
                }
                frame #4 {
                  n527 = flat-sequence {
                    frame #0 {
                      n528 = call "turn_.vi"("delay"=u32 5000, "Carzeta"=156.04) -> ()  [unwired: 10 in]
                    }
                    frame #1 {
                      n529 = expression code="x*115"(9.85) -> (w1148:dbl)
                      n530 = call "move_v2.vi"("delay"=u32 3000, "Enum"=enum16{"hold", "f", "b"}."f", "D"=w1148) -> ()  [unwired: 1 in]
                    }
                    frame #2 {
                      n531 = call "turn_.vi"("delay"=u32 1200, "Carzeta"=-23.96) -> ()  [unwired: 10 in]
                    }
                  }
                }
                frame #5 {
                  n532 = flat-sequence {
                    tunnel: [w1156] -> w1154
                    tunnel: [w1155] -> w1153
                    tunnel: w1154 -> [w1161]
                    tunnel: w1153 -> [w1160]
                    frame #0 {
                      w1155 = 0.84 ("target_ir_l")
                      w1156 = 0.84 ("target_ir_r")
                      n533 = call "integal_caribat_squence.vi"("inner_b_ir"=0.4, "inner_f_ir"=0.8, "target_ir_l"=w1155, "target_ir_r"=w1156, "precision"=0.008) -> ()
                    }
                    frame #1 {
                      n534 = call "integal_pickup_sequence .vi"("store_pos"=u8 184, "pick_pos"=u8 52, "target_ir_l"=w1160, "target_ir_r"=w1161, "precision"=0.04) -> ()
                    }
                  }
                }
                frame #6 {
                  # "154"
                  n535 = call "integal_return.vi"("servo 3 dropfront"=u8 52, "servo 3 pickBack"=u8 154) -> ()
                }
                frame #7 {
                  n536 = flat-sequence {
                    frame #0 {
                      n537 = expression code="x*115"(5.0 ("zeta")) -> (w1167:dbl)
                      n538 = call "move_.vi"("Enum"=enum16{"hold", "f", "b"}."f", "delay"=u32 5500, "D"=w1167) -> ()  [unwired: 1 in]
                    }
                    frame #1 {
                      n539 = call "turn_.vi"("delay"=u32 3000, "Carzeta"=90.0 ("zeta")) -> ()  [unwired: 10 in]
                    }
                  }
                }
                frame #8 {
                  n540 = flat-sequence {
                    tunnel: [w1176] -> w1174
                    tunnel: [w1175] -> w1173
                    tunnel: w1174 -> [w1181]
                    tunnel: w1173 -> [w1180]
                    frame #0 {
                      w1175 = 0.84 ("target_ir_l")
                      w1176 = 0.84 ("target_ir_r")
                      n541 = call "integal_caribat_squence.vi"("inner_b_ir"=0.4, "inner_f_ir"=0.8, "target_ir_l"=w1175, "target_ir_r"=w1176, "precision"=0.008) -> ()
                    }
                    frame #1 {
                      n542 = call "integal_pickup_sequence .vi"("store_pos"=u8 154, "pick_pos"=u8 52, "target_ir_l"=w1180, "target_ir_r"=w1181, "precision"=0.04) -> ()
                    }
                  }
                }
                frame #9 {
                  n543 = flat-sequence {
                    frame #0 {
                      n544 = expression code="x*115"(4.0 ("zeta")) -> (w1188:dbl)
                      n545 = call "move_.vi"("Enum"=enum16{"hold", "f", "b"}."b", "delay"=u32 4500, "D"=w1188) -> ()  [unwired: 1 in]
                    }
                    frame #1 {
                      n546 = call "turn_.vi"("delay"=u32 3000, "Carzeta"=90.0 ("zeta")) -> ()  [unwired: 10 in]
                    }
                    frame #2 {
                      # "154"
                      n547 = call "integal_return.vi"("servo 3 dropfront"=u8 52, "servo 3 pickBack"=u8 154) -> ()
                      n548 = expression code="x*115"(4.0 ("zeta")) -> (w1193:dbl)
                      n549 = call "move_.vi"("Enum"=enum16{"hold", "f", "b"}."f", "delay"=u32 4500, "D"=w1193) -> ()  [unwired: 1 in]
                    }
                  }
                }
                frame #10 {
                  n550 = flat-sequence {
                    frame #0 {
                      n551 = call "servo_pickfromback_sequence.vi"("pick_pos"=u8 182) -> ()
                    }
                    frame #1 {
                      n552 = global write "GlobalVar.vi" "servo 3"(u8 52 ("servo 3")) -> ()
                    }
                  }
                  n553 = flat-sequence {
                    frame #0 {
                      n554 = call "turn_.vi"("delay"=u32 3000, "Carzeta"=90.0 ("zeta")) -> ()  [unwired: 10 in]
                    }
                    frame #1 {
                      n555 = expression code="x*115"(1.5 ("zeta")) -> (w1204:dbl)
                      n556 = call "move_.vi"("Enum"=enum16{"hold", "f", "b"}."f", "delay"=u32 2500, "D"=w1204) -> ()  [unwired: 1 in]
                    }
                    frame #2 {
                      n557 = call "turn_.vi"("delay"=u32 3000, "Carzeta"=90.0 ("zeta")) -> ()  [unwired: 10 in]
                    }
                    frame #3 {
                      n558 = expression code="x*115"(7.5 ("zeta")) -> (w1207:dbl)
                      n559 = call "move_.vi"("Enum"=enum16{"hold", "f", "b"}."f", "delay"=u32 8000, "D"=w1207) -> ()  [unwired: 1 in]
                    }
                  }
                }
              }
            }
          }
          "binary" <- w128
        }
      }
    }
    frame Disabled {
      n560 = flat-sequence {
        frame #0 {
          n561 = global write "GlobalVar.vi" "MOTOR_POW"(i8 11 ("MOTOR_POW")) -> ()
          n562 = global write "GlobalVar.vi" "servo 3"(u8 160 ("servo 3")) -> ()
          n563 = global write "GlobalVar.vi" "servo 2"(u8 175 ("servo 2")) -> ()
          n564 = global write "GlobalVar.vi" "servo 1"(u8 160 ("servo 1")) -> ()
          n565 = global write "GlobalVar.vi" "r_wheel"(102.4 ("r_wheel")) -> ()
          n566 = global write "GlobalVar.vi" "r_car"(253.192 ("r_car")) -> ()
        }
        frame #1 {
          n567 = while {
            stop <- "done_pickup 2" stop-if-true
            n568 = flat-sequence {
              frame #0 {
                n569 = while {
                  stop <- "start_pick 2" stop-if-true
                  n570 = Wait (ms)(milliseconds to wait=u32 50) -> ()  [unwired: 1 out]
                }
              }
              frame #1 {
                n571 = local read "target_ir_r 2"() -> (w1236:dbl)
                n572 = local read "target_ir_l 2"() -> (w1237:dbl)
                n573 = call "move_to_ir.vi"("step"=2, "precision"=0.01, "target_ir_r"=w1236, "samples"=250, "delay_after"=u32 100, "target_ir_l"=w1237) -> ()
              }
              frame #2 {
                n574 = call "servo_pickfromback_sequence.vi"("pick_pos"="servo 3 pickBack 2") -> ()
              }
              frame #3 {
                n575 = call "servo_return_block_sequence.vi"("servo 3"="servo 3 dropfront 2") -> ()
              }
              frame #4 {
                n576 = global write "GlobalVar.vi" "servo 3"(u8 100 ("servo 3")) -> ()
              }
            }
          }
          n577 = while {
            stop <- "done_servo_positioning 2" stop-if-true
            n578 = flat-sequence {
              frame #0 {
                n579 = while {
                  stop <- "start_seri 2" stop-if-true
                  n580 = Wait (ms)(milliseconds to wait=u32 50) -> ()  [unwired: 1 out]
                }
              }
              frame #1 {
                n581 = local read "target_ir_r 2"() -> (w1264:dbl)
                n582 = local read "target_ir_l 2"() -> (w1263:dbl)
                n583 = call "move_to_ir.vi"("step"=2, "precision"=0.01, "target_ir_r"=w1264, "samples"=250, "delay_after"=u32 500, "target_ir_l"=w1263) -> ()
              }
              frame #2 {
                n584 = call "servo_pickup_sequence.vi"("servo 3"="servo3 pick_front 2") -> ()
              }
              frame #3 {
                n585 = call "servo_park_squence.vi"("servo 3"="servo3 drop_inBack 2") -> ()
              }
              frame #4 {
                n586 = global write "GlobalVar.vi" "servo 3"(u8 100 ("servo 3")) -> ()
              }
            }
          }
          n587 = while {
            stop <- FALSE stop-if-true
            n588 = flat-sequence {
              frame #0 {
                n589 = while {
                  stop <- "trun 2" stop-if-true
                  n590 = Wait (ms)(milliseconds to wait=u32 50) -> ()  [unwired: 1 out]
                }
              }
              frame #1 {
                n591 = flat-sequence {
                  tunnel: u32 50 ("delay_per_step") -> [w1224]
                  tunnel: "D 2" -> [w1225]
                  frame #0 {
                    n592 = call "increase_motor_pow.vi"("delay_per_step"=w1224, "max_pow"=30) -> ()
                  }
                  frame #1 {
                    n593 = expression code="x*(2)"(w1225) -> (w1226:dbl)
                    n594 = Wait (ms)(milliseconds to wait=w1226) -> ()  [unwired: 1 out]
                  }
                  frame #2 {
                    n595 = call "decrease_motor_pow.vi"("delay_per_step"=100 ("min_pow"), "min_pow"=10) -> ()
                  }
                }
                n596 = call "move_.vi"("Enum"="Enum 2", "D"="D 2") -> ()  [unwired: 2 in]
              }
              frame #2 {
              }
              frame #3 {
              }
              frame #4 {
              }
            }
          }
          n597 = while {
            stop <- "done_positioning 2" stop-if-true
            n598 = flat-sequence {
              frame #0 {
                n599 = while {
                  stop <- "start_cari 2" stop-if-true
                  n600 = Wait (ms)(milliseconds to wait=u32 50) -> ()  [unwired: 1 out]
                }
              }
              frame #1 {
                n601 = call "move_to_ir.vi"("step"=1, "precision"=0.05, "target_ir_r"="target_ir_r 2", "samples"=250, "delay_after"=u32 1000, "target_ir_l"="target_ir_l 2") -> ()
              }
              frame #2 {
                n602 = call "turn_.vi"("delay"=u32 3500, "Carzeta"=-90.0) -> ()  [unwired: 10 in]
              }
              frame #3 {
                n603 = global write "GlobalVar.vi" "MOTOR_POW"(i8 8 ("MOTOR_POW")) -> ()
              }
              frame #4 {
                n604 = call "left_centrolize_v2.vi"("samples"=200, "step(mm)"=1, "inner_b_ir"="inner_b_ir 2", "inner_f_ir"="inner_f_ir 2") -> ()
              }
              frame #5 {
                n605 = global write "GlobalVar.vi" "MOTOR_POW"(i8 11 ("MOTOR_POW")) -> ()
              }
              frame #6 {
                n606 = call "turn_.vi"("delay"=u32 2800, "Carzeta"=90.0) -> ()  [unwired: 10 in]
              }
            }
          }
        }
      }
    }
  }
  n607 = disable-structure shown="Disabled" {
    frame Disabled {
      n608 = flat-sequence {
        tunnel: [w1366] -> w1272
        tunnel: w1272 -> [w1379]
        frame #0 {
          n609 = global write "GlobalVar.vi" "MOTOR_POW"(i8 15 ("MOTOR_POW")) -> ()
          n610 = global write "GlobalVar.vi" "servo 1"(u8 160 ("servo 1")) -> ()
          n611 = global write "GlobalVar.vi" "servo 2"(u8 175 ("servo 2")) -> ()
          n612 = global write "GlobalVar.vi" "servo 3"(u8 165 ("servo 3")) -> ()
          n613 = global write "GlobalVar.vi" "r_wheel"(102.4 ("r_wheel")) -> ()
          n614 = global write "GlobalVar.vi" "r_car"(253.192 ("r_car")) -> ()
        }
        frame #1 {
          n615 = while {
            stop <- w1279 stop-if-true
            n616 = Random Number (0-1)() -> (number: 0 to 1=w1284:dbl)
            n617 = Random Number (0-1)() -> (number: 0 to 1=w1291:dbl)
            n618 = Random Number (0-1)() -> (number: 0 to 1=w1288:dbl)
            n619 = Random Number (0-1)() -> (number: 0 to 1=w1287:dbl)
            n620 = Greater?(x=w1284, y=0.5) -> (0:w1283:bool)
            n621 = Greater?(x=w1291, y=0.5) -> (0:w1282:bool)
            n622 = Greater?(x=w1288, y=0.5) -> (0:w1281:bool)
            n623 = Greater?(x=w1287, y=0.5) -> (0:w1280:bool)
            n624 = Wait (ms)(milliseconds to wait=u32 50) -> ()  [unwired: 1 out]
            n625 = xnode "Button 2"() -> ("Value"=w1279:bool)  [unwired: 1 in, 1 out]
            n626 = xnode "LED 2"("LED0"=w1283, "LED1"=w1282, "LED2"=w1281, "LED3"=w1280) -> ()  [unwired: 1 in, 1 out]
          }
        }
        frame #2 {
          n627 = flat-sequence {
            tunnel: [w1372] -> w1366
            frame #0 {
              n628 = Wait (ms)(milliseconds to wait=u32 1000) -> ()  [unwired: 1 out]
            }
            frame #1 {
              n629 = expression code="x*(2)"(115.0 ("x")) -> (w1371:dbl)
              n630 = call "move_v2.vi"("delay"=enum16{"hold", "f", "b"}."f" ("Enum"), "Enum"=u32 3000 ("delay"), "D"=w1371) -> ()  [unwired: 1 in]
            }
            frame #2 {
              n631 = call "QR Reader.vi"() -> ("eiei"=w1372:u32)
            }
          }
        }
        frame #3 {
          n632 = expression code="log2(x) +1"(w1379) -> (w1378:u32)
          n633 = case shown="8" w1379 {
            frame 0, Default {
            }
            frame 1 {
              n634 = stacked-sequence {
                frame #0 {
                  n635 = expression code="x*115"(1.5 ("x")) -> (w1418:dbl)
                  n636 = call "move_v2.vi"("delay"=enum16{"hold", "f", "b"}."f" ("Enum"), "Enum"=u32 2500 ("delay"), "D"=w1418) -> ()  [unwired: 1 in]
                }
                frame #1 {
                  n637 = call "turn_.vi"("delay"=u32 2500, "Carzeta"=-90.0) -> ()  [unwired: 10 in]
                }
                frame #2 {
                  n638 = expression code="x*115"(4.5 ("x")) -> (w1424:dbl)
                  n639 = call "move_v2.vi"("delay"=enum16{"hold", "f", "b"}."f" ("Enum"), "Enum"=u32 5000 ("delay"), "D"=w1424) -> ()  [unwired: 1 in]
                }
                frame #3 {
                  n640 = call "turn_.vi"("delay"=u32 2500, "Carzeta"=-90.0) -> ()  [unwired: 10 in]
                }
                frame #4 {
                  n641 = expression code="x*115"(10.0 ("x")) -> (w1430:dbl)
                  n642 = call "move_v2.vi"("delay"=enum16{"hold", "f", "b"}."f" ("Enum"), "Enum"=u32 12000 ("delay"), "D"=w1430) -> ()  [unwired: 1 in]
                }
                frame #5 {
                  n643 = call "turn_.vi"("delay"=u32 2500, "Carzeta"=90.0) -> ()  [unwired: 10 in]
                }
              }
            }
            frame 2 {
              n644 = stacked-sequence {
                frame #0 {
                  n645 = expression code="x*115"(1.5 ("x")) -> (w1436:dbl)
                  n646 = call "move_v2.vi"("delay"=enum16{"hold", "f", "b"}."f" ("Enum"), "Enum"=u32 2000 ("delay"), "D"=w1436) -> ()  [unwired: 1 in]
                }
                frame #1 {
                  n647 = call "turn_.vi"("delay"=u32 3000, "Carzeta"=90.0) -> ()  [unwired: 10 in]
                }
                frame #2 {
                  n648 = expression code="x*115"(5.5 ("x")) -> (w1442:dbl)
                  n649 = call "move_v2.vi"("delay"=enum16{"hold", "f", "b"}."f" ("Enum"), "Enum"=u32 6300 ("delay"), "D"=w1442) -> ()  [unwired: 1 in]
                }
                frame #3 {
                  n650 = call "turn_.vi"("delay"=u32 3000, "Carzeta"=89.0) -> ()  [unwired: 10 in]
                }
                frame #4 {
                  n651 = expression code="x*115"(8.0 ("x")) -> (w1448:dbl)
                  n652 = call "move_v2.vi"("delay"=enum16{"hold", "f", "b"}."f" ("Enum"), "Enum"=u32 10000 ("delay"), "D"=w1448) -> ()  [unwired: 1 in]
                }
              }
            }
            frame 4 {
              n653 = stacked-sequence {
                frame #0 {
                  n654 = flat-sequence {
                    tunnel: [w1460] -> w1454
                    tunnel: [w1459] -> w1452
                    tunnel: w1454 -> [w1466]
                    tunnel: [w1465] -> w1453
                    tunnel: w1452 -> [w1465]
                    tunnel: w1453 -> [w1468]
                    frame #0 {
                      n655 = expression code="x*(sqrt(5)-0.5)"(115.0 ("x")) -> (w1457:dbl)
                      n656 = call "move_v2.vi"("delay"=enum16{"hold", "f", "b"}."f" ("Enum"), "Enum"=u32 1500 ("delay"), "D"=w1457) -> ()  [unwired: 1 in]
                    }
                    frame #1 {
                      n657 = call "turn_offset.vi"("x2"=12.0, "x1"=9.0, "y2"=7.0, "y1"=6.0) -> ("dis_"=w1459:dbl, "zeta"=w1460:dbl)
                    }
                    frame #2 {
                      n658 = call "turn_.vi"("delay"=u32 2500, "Carzeta"=w1466) -> ()  [unwired: 10 in]
                    }
                    frame #3 {
                      n659 = call "move_v2.vi"("delay"=enum16{"hold", "f", "b"}."f" ("Enum"), "Enum"=u32 2000 ("delay"), "D"=w1468) -> ()  [unwired: 1 in]
                    }
                  }
                }
                frame #1 {
                  n660 = flat-sequence {
                    frame #0 {
                      n661 = call "turn_.vi"("delay"=u32 2500, "Carzeta"=90.0) -> ()  [unwired: 10 in]
                    }
                    frame #1 {
                      n662 = call "move_v2.vi"("delay"=enum16{"hold", "f", "b"}."f" ("Enum"), "Enum"=u32 0 ("delay"), "D"=57.5) -> ()  [unwired: 1 in]
                    }
                  }
                }
                frame #2 {
                  n663 = expression code="115*x"(6.0) -> (w1479:dbl)
                  n664 = call "move_v2.vi"("delay"=enum16{"hold", "f", "b"}."f" ("Enum"), "Enum"=u32 9000 ("delay"), "D"=w1479) -> ()  [unwired: 1 in]
                }
                frame #3 {
                  n665 = call "turn_.vi"("delay"=u32 3500, "Carzeta"=90.0) -> ()  [unwired: 10 in]
                }
                frame #4 {
                  n666 = expression code="115*x"(7.5) -> (w1485:dbl)
                  n667 = call "move_v2.vi"("delay"=enum16{"hold", "f", "b"}."f" ("Enum"), "Enum"=u32 8000 ("delay"), "D"=w1485) -> ()  [unwired: 1 in]
                }
              }
            }
            frame 8 {
              n668 = stacked-sequence {
                frame #0 {
                  n669 = flat-sequence {
                    tunnel: [w1494] -> w1488
                    tunnel: [w1493] -> w1486
                    tunnel: w1488 -> [w1500]
                    tunnel: [w1502] -> w1487
                    tunnel: w1486 -> [w1502]
                    tunnel: w1487 -> [w1504]
                    frame #0 {
                      n670 = expression code="x*(sqrt(5)-0.5)"(115.0 ("x")) -> (w1491:dbl)
                      n671 = call "move_v2.vi"("delay"=enum16{"hold", "f", "b"}."f" ("Enum"), "Enum"=u32 1500 ("delay"), "D"=w1491) -> ()  [unwired: 1 in]
                    }
                    frame #1 {
                      n672 = call "turn_offset.vi"("x2"=13.0, "x1"=12.0, "y2"=13.0, "y1"=11.0) -> ("dis_"=w1493:dbl, "zeta"=w1494:dbl)
                    }
                    frame #2 {
                      n673 = expression code="90-x"(w1500) -> (w1499:dbl)
                      n674 = Negate(x=w1499) -> (-x=w1501:dbl)
                      n675 = call "turn_.vi"("delay"=u32 2500, "Carzeta"=w1501) -> ()  [unwired: 10 in]
                    }
                    frame #3 {
                      n676 = call "move_v2.vi"("delay"=enum16{"hold", "f", "b"}."f" ("Enum"), "Enum"=u32 2000 ("delay"), "D"=w1504) -> ()  [unwired: 1 in]
                    }
                  }
                }
                frame #1 {
                  n677 = flat-sequence {
                    frame #0 {
                      n678 = call "turn_.vi"("delay"=u32 3000, "Carzeta"=-90.0) -> ()  [unwired: 10 in]
                    }
                    frame #1 {
                      n679 = call "move_v2.vi"("delay"=enum16{"hold", "f", "b"}."f" ("Enum"), "Enum"=u32 0 ("delay"), "D"=0.0) -> ()  [unwired: 1 in]
                    }
                  }
                }
                frame #2 {
                  n680 = expression code="115*x"(5.0) -> (w1515:dbl)
                  n681 = call "move_v2.vi"("delay"=enum16{"hold", "f", "b"}."f" ("Enum"), "Enum"=u32 6500 ("delay"), "D"=w1515) -> ()  [unwired: 1 in]
                }
                frame #3 {
                  n682 = call "turn_.vi"("delay"=u32 3000, "Carzeta"=-90.0) -> ()  [unwired: 10 in]
                }
                frame #4 {
                  n683 = expression code="115*x"(6.5) -> (w1521:dbl)
                  n684 = call "move_v2.vi"("delay"=enum16{"hold", "f", "b"}."f" ("Enum"), "Enum"=u32 8000 ("delay"), "D"=w1521) -> ()  [unwired: 1 in]
                }
                frame #5 {
                  n685 = flat-sequence {
                    frame #0 {
                      n686 = call "turn_.vi"("delay"=u32 3000, "Carzeta"=90.0) -> ()  [unwired: 10 in]
                    }
                  }
                }
              }
            }
            frame 16 {
              n687 = stacked-sequence {
                frame #0 {
                  n688 = flat-sequence {
                    tunnel: [w1532] -> w1525
                    tunnel: [w1531] -> w1524
                    tunnel: [w1538] -> w1526
                    tunnel: w1525 -> [w1538]
                    tunnel: w1524 -> [w1537]
                    tunnel: w1526 -> [w1540]
                    frame #0 {
                      n689 = expression code="x*(sqrt(5)-0.5)"(115.0 ("x")) -> (w1529:dbl)
                      n690 = call "move_v2.vi"("delay"=enum16{"hold", "f", "b"}."f" ("Enum"), "Enum"=u32 1500 ("delay"), "D"=w1529) -> ()  [unwired: 1 in]
                    }
                    frame #1 {
                      n691 = call "turn_offset.vi"("x2"=12.0, "x1"=10.0, "y2"=15.0, "y1"=16.0) -> ("dis_"=w1532:dbl, "zeta"=w1531:dbl)
                    }
                    frame #2 {
                      n692 = call "turn_.vi"("delay"=u32 1000, "Carzeta"=w1537) -> ()  [unwired: 10 in]
                    }
                    frame #3 {
                      n693 = call "move_v2.vi"("delay"=enum16{"hold", "f", "b"}."f" ("Enum"), "Enum"=u32 1500 ("delay"), "D"=w1540) -> ()  [unwired: 1 in]
                    }
                  }
                }
                frame #1 {
                  n694 = flat-sequence {
                    frame #0 {
                      n695 = call "turn_.vi"("delay"=u32 3000, "Carzeta"=90.0) -> ()  [unwired: 10 in]
                    }
                    frame #1 {
                      n696 = call "move_v2.vi"("delay"=enum16{"hold", "f", "b"}."f" ("Enum"), "Enum"=u32 0 ("delay"), "D"=50.0) -> ()  [unwired: 1 in]
                    }
                  }
                }
                frame #2 {
                  n697 = expression code="115*x"(6.0) -> (w1551:dbl)
                  n698 = call "move_v2.vi"("delay"=enum16{"hold", "f", "b"}."f" ("Enum"), "Enum"=u32 7000 ("delay"), "D"=w1551) -> ()  [unwired: 1 in]
                }
                frame #3 {
                  n699 = call "turn_.vi"("delay"=u32 2500, "Carzeta"=90.0) -> ()  [unwired: 10 in]
                }
                frame #4 {
                  n700 = expression code="115*x"(1.0) -> (w1557:dbl)
                  n701 = call "move_v2.vi"("delay"=enum16{"hold", "f", "b"}."f" ("Enum"), "Enum"=u32 1500 ("delay"), "D"=w1557) -> ()  [unwired: 1 in]
                }
                frame #5 {
                  n702 = flat-sequence {
                    frame #0 {
                      n703 = call "turn_.vi"("delay"=u32 3000, "Carzeta"=-90.0) -> ()  [unwired: 10 in]
                    }
                  }
                }
              }
            }
          }
          n704 = Number To Boolean Array(number=w1378) -> (Boolean array=w1377:bool[])
          n705 = Index Array(array=w1377) -> (element #1=w1376:bool, element #2=w1375:bool, element #3=w1374:bool, element #4=w1373:bool)  [unwired: 4 in]
          n706 = xnode "LED 4"("LED0"=w1376, "LED1"=w1375, "LED2"=w1374, "LED3"=w1373) -> ()  [unwired: 1 in, 1 out]
        }
        frame #4 {
          n707 = call "move_to_ir.vi"("step"=1, "precision"=0.01, "target_ir_r"=0.845, "samples"=250, "delay_after"=u32 1000, "target_ir_l"=0.85 ("target_ir_r")) -> ()
        }
        frame #5 {
          n708 = call "turn_.vi"("delay"=u32 3000, "Carzeta"=-90.0) -> ()  [unwired: 10 in]
        }
        frame #6 {
          n709 = call "left_side_centralize.vi"("samples"=250, "step(mm)"=1, "inner_b_ir"=0.4, "inner_f_ir"=0.75) -> ()
        }
        frame #7 {
          n710 = call "attack.vi"() -> ()  [unwired: 12 in]
          n711 = call "turn_.vi"("delay"=u32 3000, "Carzeta"=90.0) -> ()  [unwired: 10 in]
        }
      }
    }
    frame Enabled {
    }
  }
  n712 = disable-structure shown="Disabled" {
    frame Disabled {
      n713 = flat-sequence {
        frame #0 {
          n714 = global write "GlobalVar.vi" "MOTOR_POW"(i8 11 ("MOTOR_POW")) -> ()
          n715 = global write "GlobalVar.vi" "servo 1"(u8 160 ("servo 1")) -> ()
          n716 = global write "GlobalVar.vi" "servo 2"(u8 190 ("servo 2")) -> ()
          n717 = global write "GlobalVar.vi" "servo 3"(u8 165 ("servo 3")) -> ()
          n718 = global write "GlobalVar.vi" "r_wheel"(102.4 ("r_wheel")) -> ()
          n719 = global write "GlobalVar.vi" "r_car"(253.192 ("r_car")) -> ()
        }
        frame #1 {
          n720 = while {
            stop <- "start_step_for_takePic" stop-if-true
            n721 = Random Number (0-1)() -> (number: 0 to 1=w1585:dbl)
            n722 = Random Number (0-1)() -> (number: 0 to 1=w1592:dbl)
            n723 = Random Number (0-1)() -> (number: 0 to 1=w1589:dbl)
            n724 = Random Number (0-1)() -> (number: 0 to 1=w1588:dbl)
            n725 = Greater?(x=w1585, y=0.5) -> (0:w1584:bool)
            n726 = Greater?(x=w1592, y=0.5) -> (0:w1583:bool)
            n727 = Greater?(x=w1589, y=0.5) -> (0:w1582:bool)
            n728 = Greater?(x=w1588, y=0.5) -> (0:w1581:bool)
            n729 = Wait (ms)(milliseconds to wait=u32 50) -> ()  [unwired: 1 out]
            n730 = xnode "LED 3"("LED0"=w1584, "LED1"=w1583, "LED2"=w1582, "LED3"=w1581) -> ()  [unwired: 1 in, 1 out]
          }
        }
        frame #2 {
          n731 = flat-sequence {
            frame #0 {
              n732 = Wait (ms)(milliseconds to wait=u32 1000) -> ()  [unwired: 1 out]
            }
            frame #1 {
              n733 = expression code="x*115"("x") -> (w1636:dbl)
              n734 = call "move_v2.vi"("delay"=enum16{"hold", "f", "b"}."b" ("Enum"), "Enum"=u32 3000 ("delay"), "D"=w1636) -> ()  [unwired: 1 in]
            }
            frame #2 {
            }
          }
        }
        frame #3 {
          n735 = while {
            stop <- FALSE stop-if-true
            n736 = flat-sequence {
              frame #0 {
                n737 = while {
                  stop <- "start_rotate_for_takePic" stop-if-true
                }
              }
              frame #1 {
                n738 = call "turn_.vi"("Carzeta"="Carzeta") -> ()  [unwired: 11 in]
              }
            }
            n739 = Wait (ms)(milliseconds to wait=u32 10) -> ()  [unwired: 1 out]
          }
        }
        frame #4 {
        }
        frame #5 {
        }
        frame #6 {
        }
        frame #7 {
        }
        frame #8 {
        }
      }
    }
    frame Enabled {
    }
  }
  n740 = disable-structure shown="Disabled" {
    frame Disabled {
      n741 = flat-sequence {
        frame #0 {
          n742 = global write "GlobalVar.vi" "MOTOR_POW"(i8 11 ("MOTOR_POW")) -> ()
          n743 = global write "GlobalVar.vi" "servo 1"(u8 160 ("servo 1")) -> ()
          n744 = global write "GlobalVar.vi" "servo 2"(u8 190 ("servo 2")) -> ()
          n745 = global write "GlobalVar.vi" "servo 3"(u8 100 ("servo 3")) -> ()
          n746 = global write "GlobalVar.vi" "r_wheel"(102.4 ("r_wheel")) -> ()
          n747 = global write "GlobalVar.vi" "r_car"(253.192 ("r_car")) -> ()
        }
        frame #1 {
          n748 = Wait (ms)(milliseconds to wait=u32 3000) -> ()  [unwired: 1 out]
        }
        frame #2 {
          n749 = call "move_to_ir.vi"("step"=1, "precision"=0.008, "target_ir_r"=0.85, "samples"=3000, "delay_after"=u32 1000, "target_ir_l"=0.85 ("target_ir_r")) -> ()
        }
        frame #3 {
          n750 = call "turn_.vi"("delay"=u32 3000, "Carzeta"=-90.0) -> ()  [unwired: 10 in]
        }
        frame #4 {
          n751 = call "left_side_centralize.vi"("samples"=3000, "step(mm)"=2, "inner_b_ir"=0.45, "inner_f_ir"=0.7) -> ()
        }
        frame #5 {
          n752 = call "servo_pickup_sequence.vi"("servo 3"=u8 38) -> ()
          n753 = call "turn_.vi"("delay"=u32 3000, "Carzeta"=90.0) -> ()  [unwired: 10 in]
        }
        frame #6 {
          # "r = 165 , l =144 | 160"
          n754 = call "servo_park_squence.vi"("servo 3"=u8 165) -> ()
        }
        frame #7 {
        }
      }
    }
    frame Enabled {
    }
  }
  n755 = disable-structure shown="Disabled" {
    frame Disabled {
      n756 = flat-sequence {
        frame #0 {
          n757 = global write "GlobalVar.vi" "MOTOR_POW"(i8 11 ("MOTOR_POW")) -> ()
          n758 = global write "GlobalVar.vi" "servo 2"(u8 190 ("servo 2")) -> ()
          n759 = global write "GlobalVar.vi" "servo 3"(u8 100 ("servo 3")) -> ()
          n760 = global write "GlobalVar.vi" "servo 1"(u8 160 ("servo 1")) -> ()
          n761 = global write "GlobalVar.vi" "r_wheel"(102.4 ("r_wheel")) -> ()
          n762 = global write "GlobalVar.vi" "r_car"(253.192 ("r_car")) -> ()
        }
        frame #1 {
          n763 = Wait (ms)(milliseconds to wait=u32 1500) -> ()  [unwired: 1 out]
        }
        frame #2 {
          w1675 = 0.85 ("target_ir_r")
          n764 = call "move_to_ir.vi"("step"=2, "precision"=0.005, "target_ir_r"=w1675, "samples"=3000, "delay_after"=u32 1000, "target_ir_l"=w1675) -> ()
        }
        frame #3 {
          # "r = 165 , l =144 | 160"
          n765 = flat-sequence {
            frame #0 {
              n766 = call "turn_.vi"("delay"=u32 2500, "Carzeta"=-90.0) -> ()  [unwired: 10 in]
            }
            frame #1 {
              n767 = call "left_side_centralize.vi"("samples"=3000, "step(mm)"=2, "inner_b_ir"=0.4, "inner_f_ir"=0.7) -> ()
            }
            frame #2 {
              n768 = call "turn_.vi"("delay"=u32 3000, "Carzeta"=90.0) -> ()  [unwired: 10 in]
            }
          }
          n769 = call "servo_pickfromback_sequence.vi"("pick_pos"=u8 159 ("servo 3")) -> ()
        }
        frame #4 {
        }
        frame #5 {
        }
        frame #6 {
        }
        frame #7 {
        }
      }
    }
    frame Enabled {
    }
  }
  n770 = disable-structure shown="Disabled" {
    frame Disabled {
      n771 = flat-sequence {
        frame #0 {
          n772 = global write "GlobalVar.vi" "MOTOR_POW"(i8 11 ("MOTOR_POW")) -> ()
          n773 = global write "GlobalVar.vi" "servo 1"(u8 160 ("servo 1")) -> ()
          n774 = global write "GlobalVar.vi" "servo 2"(u8 175 ("servo 2")) -> ()
          n775 = global write "GlobalVar.vi" "servo 3"(u8 160 ("servo 3")) -> ()
          n776 = global write "GlobalVar.vi" "r_wheel"(102.4 ("r_wheel")) -> ()
          n777 = global write "GlobalVar.vi" "r_car"(253.192 ("r_car")) -> ()
        }
        frame #1 {
          n778 = while {
            stop <- "done_servo_positioning" stop-if-true
            n779 = flat-sequence {
              frame #0 {
                n780 = while {
                  stop <- "start_seri" stop-if-true
                  n781 = Wait (ms)(milliseconds to wait=u32 50) -> ()  [unwired: 1 out]
                }
              }
              frame #1 {
                n782 = local read "target_ir_r"() -> (w1738:dbl)
                n783 = local read "target_ir_l"() -> (w1737:dbl)
                n784 = call "move_to_ir.vi"("step"=2, "precision"=0.01, "target_ir_r"=w1738, "samples"=250, "delay_after"=u32 500, "target_ir_l"=w1737) -> ()
              }
              frame #2 {
                n785 = call "servo_pickup_sequence.vi"("servo 3"="servo3 pick_front") -> ()
              }
              frame #3 {
                n786 = call "servo_park_squence.vi"("servo 3"="servo3 drop_inBack") -> ()
              }
              frame #4 {
                n787 = global write "GlobalVar.vi" "servo 3"(u8 100 ("servo 3")) -> ()
              }
            }
          }
          n788 = while {
            stop <- "done_positioning" stop-if-true
            n789 = flat-sequence {
              frame #0 {
                n790 = while {
                  stop <- "start_cari" stop-if-true
                  n791 = Wait (ms)(milliseconds to wait=u32 50) -> ()  [unwired: 1 out]
                }
              }
              frame #1 {
                n792 = call "move_to_ir.vi"("step"=1, "precision"=0.05, "target_ir_r"="target_ir_r", "samples"=250, "delay_after"=u32 1000, "target_ir_l"="target_ir_l") -> ()
              }
              frame #2 {
                n793 = call "turn_.vi"("delay"=u32 3500, "Carzeta"=-90.0) -> ()  [unwired: 10 in]
              }
              frame #3 {
                n794 = global write "GlobalVar.vi" "MOTOR_POW"(i8 8 ("MOTOR_POW")) -> ()
              }
              frame #4 {
                n795 = call "left_centrolize_v2.vi"("samples"=200, "step(mm)"=1, "inner_b_ir"="inner_b_ir", "inner_f_ir"="inner_f_ir") -> ()
              }
              frame #5 {
                n796 = global write "GlobalVar.vi" "MOTOR_POW"(i8 11 ("MOTOR_POW")) -> ()
              }
              frame #6 {
                n797 = call "turn_.vi"("delay"=u32 2800, "Carzeta"=90.0) -> ()  [unwired: 10 in]
              }
            }
          }
          n798 = while {
            stop <- "done_pickup" stop-if-true
            n799 = flat-sequence {
              frame #0 {
                n800 = while {
                  stop <- "start_pick" stop-if-true
                  n801 = Wait (ms)(milliseconds to wait=u32 50) -> ()  [unwired: 1 out]
                }
              }
              frame #1 {
                n802 = local read "target_ir_r"() -> (w1710:dbl)
                n803 = local read "target_ir_l"() -> (w1711:dbl)
                n804 = call "move_to_ir.vi"("step"=2, "precision"=0.01, "target_ir_r"=w1710, "samples"=250, "delay_after"=u32 100, "target_ir_l"=w1711) -> ()
              }
              frame #2 {
                n805 = call "servo_pickfromback_sequence.vi"("pick_pos"="servo 3 pickBack") -> ()
              }
              frame #3 {
                n806 = call "servo_return_block_sequence.vi"("servo 3"="servo 3 dropfront") -> ()
              }
              frame #4 {
                n807 = global write "GlobalVar.vi" "servo 3"(u8 100 ("servo 3")) -> ()
              }
            }
          }
          n808 = while {
            stop <- FALSE stop-if-true
            n809 = flat-sequence {
              frame #0 {
                n810 = while {
                  stop <- "trun" stop-if-true
                  n811 = Wait (ms)(milliseconds to wait=u32 50) -> ()  [unwired: 1 out]
                }
              }
              frame #1 {
                n812 = flat-sequence {
                  tunnel: u32 50 ("delay_per_step") -> [w1698]
                  tunnel: "D" -> [w1699]
                  frame #0 {
                    n813 = call "increase_motor_pow.vi"("delay_per_step"=w1698, "max_pow"=30) -> ()
                  }
                  frame #1 {
                    n814 = expression code="x*(2)"(w1699) -> (w1700:dbl)
                    n815 = Wait (ms)(milliseconds to wait=w1700) -> ()  [unwired: 1 out]
                  }
                  frame #2 {
                    n816 = call "decrease_motor_pow.vi"("delay_per_step"=100 ("min_pow"), "min_pow"=10) -> ()
                  }
                }
                n817 = call "move_.vi"("Enum"="Enum", "D"="D") -> ()  [unwired: 2 in]
              }
              frame #2 {
              }
              frame #3 {
              }
              frame #4 {
              }
            }
          }
        }
      }
    }
    frame Enabled {
    }
  }
  n818 = while {
    stop <- FALSE stop-if-true
    n819 = disable-structure shown="Disabled" {
      frame Disabled {
        n820 = call "Vision Acquisition"("Stop (F)"="Stop (F)") -> ("Image Out"=→"Image Out":T1)  [unwired: 24 in, 2 out]
      }
      frame Enabled {
      }
    }
    n821 = global read "GlobalVar.vi" "servo 3"() -> (w1753:u8)
    n822 = global read "GlobalVar.vi" "L_MOTOR_POS"() -> (w1747:i32)
    "L_MOTOR_POS" <- w1747
    n823 = global read "GlobalVar.vi" "R_MOTOR_POS"() -> (w1746:i32)
    "R_MOTOR_POS" <- w1746
    n824 = global read "GlobalVar.vi" "MOTOR_POW"() -> (w1748:i8)
    "MOTOR_POW" <- w1748
    n825 = case shown="1, Default" w1753 {
      frame 0 {
      }
      frame 1, Default {
        n826 = global read "GlobalVar.vi" "servo 1"() -> (w1758:u8)
        n827 = global read "GlobalVar.vi" "servo 2"() -> (w1757:u8)
        n828 = global read "GlobalVar.vi" "servo 3"() -> (w1756:u8)
        n829 = call <vilib>:"TETRIX Servos Move All_HT_myRIO.vi"("Enable Sync: Fast | Medium | Slow | None"="Medium", "Controller Daisy Chain Position (1 - 4)"=u8 2, "Servo 3 (0 - 255)"=w1756, "Servo 2 (0 - 255)"=w1757, "Servo 1 (0 - 255)"=w1758) -> ()  [unwired: 4 in, 1 out]
      }
    }
    n830 = call <vilib>:"TETRIX Motor(s) Move_HT_myRIO.vi"("Motor 2 Power (-100 to 100)\n0 = Stop/Brake\n-128 = Stop/Coast"=w1748, "Motor 1 Power (-100 to 100)\n0 = Stop/Brake\n-128 = Stop/Coast"=w1748, "Control Mode"="Run to Position", "Motor 2 Reverse? : T or F"=TRUE, "Motor 1 Reverse? : T or F"=FALSE, "Encoder 2 Target: 360 = 1 motor shaft revolution"=w1746, "Encoder 1 Target: 360 = 1 motor shaft revolution"=w1747, "Controller Daisy Chain Position: 1 - 4"=u8 1) -> ()  [unwired: 1 in, 1 out]
    n831 = Wait (ms)(milliseconds to wait=u32 0) -> ()  [unwired: 1 out]
  }
